vi "ACT_Loop.vi"() -> ()   [LabVIEW 2023, in "Swerve-SteerSRX-DriveSpark-AbsAnalog_ACT.lvlib"]
uses:
  Swerve-SteerSRX-DriveSpark-AbsAnalog_ACT.lvlib
  Cluster_CMD_ACT_Data.ctl
  ENUM_CMD_Mode Select.ctl
  Shared Code/TypeDefs/Cluster_CMD_Direction Data.ctl
  Shared Code/TypeDefs/Cluster_Module Velocity-Direction-Rotations.ctl
  Shared Code/TypeDefs/Level_Velocity plus-minus 1.ctl
  Shared Code/TypeDefs/Dial_Compase heading unit circle CCW positive.ctl
  Shared Code/TypeDefs/Cluster_X-Y.ctl
  Cluster_HW Output Values.ctl
  Shared Code/TypeDefs/Cluster_Swerve 4 Steer and Velocity.ctl
  Cluster_System Output Data.ctl
  Cluster_System Config_Values.ctl
  Shared Code/TypeDefs/Cluster_SW PID Config.ctl
  Shared Code/TypeDefs/Cluster_PID Gains.ctl
  Shared Code/TypeDefs/Cluster_High-Low.ctl
  Type Defs/Cluster_Length and Width.ctl
  Shared Code/TypeDefs/Cluster_Config_Swerve_Drive Param.ctl
  Shared Code/TypeDefs/Cluster_Config_Swerve_Steer Parm.ctl
  Cluster_Config Specific HW Values.ctl
  Cluster_Config Specific Data.ctl
  Shared Code/TypeDefs/ENUM_Module Position.ctl
  Cluster_Config Steer HW Values.ctl
  Shared Code/TypeDefs/Cluster_Config SRX Motor Output.ctl
  <vilib>/Rock Robotics/WPI/ThirdParty/Phoenix-LabVIEW/Motor Controller/Controls/CTRE_Phoenix_MotorControl_NeutralMode.ctl
  Shared Code/TypeDefs/Cluster_FWD  REV Values.ctl
  Shared Code/TypeDefs/Cluster_SRX SLOT PID Config.ctl
  Shared Code/TypeDefs/Cluster_SRX Motion Magic Parameters.ctl
  Cluster_Config Drive HW Values.ctl
  Shared Code/TypeDefs/Cluster_SparkMax Config_Motor Output.ctl
  <vilib>/Rock Robotics/WPI/ThirdParty/REV Robotics/REVLib/Typedef/Spark MAX Idle Mode.ctl
  Shared Code/TypeDefs/Cluster_Spark MAX Config_SLOT PID Config.ctl
  Shared Code/TypeDefs/Cluster_SparkMax Config_Smart Motion Parameters.ctl
  ENUM_ACT_State.ctl
  <vilib>/Rock Robotics/WPI/ThirdParty/Phoenix-LabVIEW/Motor Controller/Controls/CTRE_Phoenix_MotorControl_ControlMode.ctl
  <vilib>/Rock Robotics/WPI/MotorControl/WPI_MotorControlDeviceRef.ctl
  <vilib>/Rock Robotics/WPI/MotorControl/WPI_MotorControlType.ctl
  <vilib>/Rock Robotics/SystemInterfaces/DIO/FPGA_DIOPWMChannel.ctl
  <vilib>/Rock Robotics/WPI/PWM/WPI_PWMDeadband.ctl
  <vilib>/Rock Robotics/SystemInterfaces/DIO/FPGA_DIOChannel.ctl
  ENUM_ACT_Action.ctl
  4f1f8321-3dc8-4b28-8619-20673fc77ec2.vi
  cbff3d61-3b62-444e-9844-795ae03579cd.vi
  089052c0-d540-4a78-a5cc-aeb70dbb496b.vi
  6201c2b1-dcd8-4430-86f1-9b4ee56c7753.vi
  b5508d6c-c1cc-4273-80c5-2077d34e1483.vi
  5f725c2a-0ce1-4524-8967-e83b15fdce90.vi
  bd5da564-2e8e-4505-86fc-30918feadaa2.vi
  8beda75f-c59a-4462-acc7-7c37ceab3777.vi
  47a9b741-f4a3-48b6-ae85-4ba2e502368e.vi
  e2e8a241-7810-4d95-85fd-17f3a55957a8.vi
  80d407e5-f582-430c-986f-ecd413765478.vi
  573e44c0-11f4-4bd9-ad56-904ec25dba75.vi
  e7494af9-f670-4352-9dfa-ae6ce50709ea.vi
  <vilib>/Utility/error.llb/Trim Whitespace.vi
  5f725c2a-0ce1-4524-8967-e83b15fdce90.vi/958b2683-dd4b-41b7-8ed1-41c95f63cef0.vi
  5f725c2a-0ce1-4524-8967-e83b15fdce90.vi/95f5fa9b-6175-4b34-88ee-cece92c38279.vi
  bd5da564-2e8e-4505-86fc-30918feadaa2.vi/958b2683-dd4b-41b7-8ed1-41c95f63cef0.vi
  bd5da564-2e8e-4505-86fc-30918feadaa2.vi/95f5fa9b-6175-4b34-88ee-cece92c38279.vi
  8beda75f-c59a-4462-acc7-7c37ceab3777.vi/958b2683-dd4b-41b7-8ed1-41c95f63cef0.vi
  8beda75f-c59a-4462-acc7-7c37ceab3777.vi/95f5fa9b-6175-4b34-88ee-cece92c38279.vi
  47a9b741-f4a3-48b6-ae85-4ba2e502368e.vi/958b2683-dd4b-41b7-8ed1-41c95f63cef0.vi
  47a9b741-f4a3-48b6-ae85-4ba2e502368e.vi/95f5fa9b-6175-4b34-88ee-cece92c38279.vi
  e2e8a241-7810-4d95-85fd-17f3a55957a8.vi/958b2683-dd4b-41b7-8ed1-41c95f63cef0.vi
  e2e8a241-7810-4d95-85fd-17f3a55957a8.vi/95f5fa9b-6175-4b34-88ee-cece92c38279.vi
  80d407e5-f582-430c-986f-ecd413765478.vi/958b2683-dd4b-41b7-8ed1-41c95f63cef0.vi
  80d407e5-f582-430c-986f-ecd413765478.vi/95f5fa9b-6175-4b34-88ee-cece92c38279.vi
  573e44c0-11f4-4bd9-ad56-904ec25dba75.vi/958b2683-dd4b-41b7-8ed1-41c95f63cef0.vi
  573e44c0-11f4-4bd9-ad56-904ec25dba75.vi/95f5fa9b-6175-4b34-88ee-cece92c38279.vi
  e7494af9-f670-4352-9dfa-ae6ce50709ea.vi/958b2683-dd4b-41b7-8ed1-41c95f63cef0.vi
  e7494af9-f670-4352-9dfa-ae6ce50709ea.vi/95f5fa9b-6175-4b34-88ee-cece92c38279.vi
  <vilib>/Utility/error.llb/Trim Whitespace One-Sided.vi
  5f725c2a-0ce1-4524-8967-e83b15fdce90.vi/95f5fa9b-6175-4b34-88ee-cece92c38279.vi/1c6bd52c-bbca-4d4a-a290-93ea2703fded.vi
  5f725c2a-0ce1-4524-8967-e83b15fdce90.vi/95f5fa9b-6175-4b34-88ee-cece92c38279.vi/47c2b0d5-b5fa-444e-9535-611565d375db.vi
  bd5da564-2e8e-4505-86fc-30918feadaa2.vi/95f5fa9b-6175-4b34-88ee-cece92c38279.vi/1c6bd52c-bbca-4d4a-a290-93ea2703fded.vi
  bd5da564-2e8e-4505-86fc-30918feadaa2.vi/95f5fa9b-6175-4b34-88ee-cece92c38279.vi/47c2b0d5-b5fa-444e-9535-611565d375db.vi
  8beda75f-c59a-4462-acc7-7c37ceab3777.vi/95f5fa9b-6175-4b34-88ee-cece92c38279.vi/1c6bd52c-bbca-4d4a-a290-93ea2703fded.vi
  8beda75f-c59a-4462-acc7-7c37ceab3777.vi/95f5fa9b-6175-4b34-88ee-cece92c38279.vi/47c2b0d5-b5fa-444e-9535-611565d375db.vi
  47a9b741-f4a3-48b6-ae85-4ba2e502368e.vi/95f5fa9b-6175-4b34-88ee-cece92c38279.vi/1c6bd52c-bbca-4d4a-a290-93ea2703fded.vi
  47a9b741-f4a3-48b6-ae85-4ba2e502368e.vi/95f5fa9b-6175-4b34-88ee-cece92c38279.vi/47c2b0d5-b5fa-444e-9535-611565d375db.vi
  e2e8a241-7810-4d95-85fd-17f3a55957a8.vi/95f5fa9b-6175-4b34-88ee-cece92c38279.vi/1c6bd52c-bbca-4d4a-a290-93ea2703fded.vi
  e2e8a241-7810-4d95-85fd-17f3a55957a8.vi/95f5fa9b-6175-4b34-88ee-cece92c38279.vi/47c2b0d5-b5fa-444e-9535-611565d375db.vi
  80d407e5-f582-430c-986f-ecd413765478.vi/95f5fa9b-6175-4b34-88ee-cece92c38279.vi/1c6bd52c-bbca-4d4a-a290-93ea2703fded.vi
  80d407e5-f582-430c-986f-ecd413765478.vi/95f5fa9b-6175-4b34-88ee-cece92c38279.vi/47c2b0d5-b5fa-444e-9535-611565d375db.vi
  573e44c0-11f4-4bd9-ad56-904ec25dba75.vi/95f5fa9b-6175-4b34-88ee-cece92c38279.vi/1c6bd52c-bbca-4d4a-a290-93ea2703fded.vi
  573e44c0-11f4-4bd9-ad56-904ec25dba75.vi/95f5fa9b-6175-4b34-88ee-cece92c38279.vi/47c2b0d5-b5fa-444e-9535-611565d375db.vi
  e7494af9-f670-4352-9dfa-ae6ce50709ea.vi/95f5fa9b-6175-4b34-88ee-cece92c38279.vi/1c6bd52c-bbca-4d4a-a290-93ea2703fded.vi
  e7494af9-f670-4352-9dfa-ae6ce50709ea.vi/95f5fa9b-6175-4b34-88ee-cece92c38279.vi/47c2b0d5-b5fa-444e-9535-611565d375db.vi
  RoboRIO Utilities/Global_STOP.vi
  Global_CMD_ACT_Data In.vi
  PigeonIMU/Global_SEN_Data Out.vi
  Global_ACT_Data Out.vi
  <vilib>/Utility/Data Type/Get Type Information.vi
  Shared Code/Utility/RWA/RWA/File/RWA_PC FIle Read String.vi
  Shared Code/Utility/RWA/RWA/Read Write Anything/RWA_File String.vi
  Shared Code/Utility/RWA/RWA/File/RWA_PC File Write String.vi
  <vilib>/Comparison/Equal/Equal Functor/Equal Functor.lvclass
  PigeonIMU/PigeonIMU_SEN_ts.lvlib
panel:
  in  "Set Steer Start Values":bool
  in  "Config Drive":T1={"Drive HW Ver"=0, "SparkMax Output"={"Motor Invert"=FALSE, "Ramp Rate OL (S)"=1.0, "Dead Band"=0.0, "Idle Mode"=enum."Coast"}, "Slot 0 CL"={"Gains"={"P"=0.1, "I"=0.0, "D"=0.0, "F"=0.0}, "I Zone"=0.0, "Peak Out -1 0 1"={"High"=0.0, "Low"=0.0}, "Max I Accu"=0.0}, "Slot 0 SM"={"Max Velocity"=0.0, "Max Acceleration"=0.0, "Allowed CL Error"=0.0, "Min Velocity Output"=0.0}} {"Slot 0 CL"."Gains"."F" format="%#.8f"; "Slot 0 CL"."Gains"."D" format="%#.8f"; "Slot 0 CL"."Gains"."I" format="%#.8f"; "Slot 0 CL"."Gains"."P" format="%#.8f"; "Slot 0 CL"."Peak Out -1 0 1"."Low" format="%#.8f"; "Slot 0 CL"."Peak Out -1 0 1"."High" format="%#.8f"}
  in  "Config Steer":T8={"Steer HW Ver"=0, "SRX Output"={"Neutral"=enum."Override to Coast", "Max"={"FWD"=1.0, "REV"=-1.0}, "Min"={"FWD"=0.0, "REV"=0.0}, "OL Ramp Rate (S)"=0.0, "Dead Band"=0.0, "CL Ramp Rate (S)"=0.0}, "Slot 0 CL"={"Gains"={"P"=1.0, "I"=0.01, "D"=0.0, "F"=0.0}, "Error Allowed"=0.0, "I Zone"=10000.0, "Peak Out 0-1"=1.0, "Max I Accu"=-1000.0}, "Slot 0 MM"={"Cruise Velocity"=5000, "Acceleration"=5000}} {"Slot 0 CL"."Gains"."F" format="%#.8f"; "Slot 0 CL"."Gains"."D" format="%#.8f"; "Slot 0 CL"."Gains"."I" format="%#.8f"; "Slot 0 CL"."Gains"."P" format="%#.8f"; "SRX Output"."Min"."REV" format="%.2f"; "SRX Output"."Min"."FWD" format="%.2f"; "SRX Output"."Max"."REV" format="%.2f"; "SRX Output"."Max"."FWD" format="%.2f"}
  in  "Config Specific":T14={"Specific HW Ver"=0, "Specific Data"=[{"Motor Pos"=enum."Left-Front", "CAN Bus"="", "Drive ID"=0, "Steer ID"=0, "Encoder Start Value"=0.0}, {"Motor Pos"=enum."Right-Front", "CAN Bus"="", "Drive ID"=0, "Steer ID"=0, "Encoder Start Value"=0.0}, {"Motor Pos"=enum."Right-Back", "CAN Bus"="", "Drive ID"=0, "Steer ID"=0, "Encoder Start Value"=0.0}, {"Motor Pos"=enum."Left-Back", "CAN Bus"="", "Drive ID"=0, "Steer ID"=0, "Encoder Start Value"=0.0}]}
  in  "CMD Override":enum32{"None", "Mode 2", "Mode 1", "STOP"}(tab)
  in  "Mode 2 Data":dbl(slide) scale=-0.2..0.2
  in  "Mode 1 Data":i32
  in  "GO":bool
  out "Current Time":timestamp
  in  "Config System":T17={"System Ver"=0, "Auto Angle PID"={"Gains"={"P"=0.1, "I"=0.0, "D"=0.0, "F"=0.0}, "Error Allowed"={"High"=0.0, "Low"=0.0}, "I Zone"={"High"=0.0, "Low"=0.0}, "Peak Out 0-1"={"High"=0.0, "Low"=0.0}, "Max I Accu"={"High"=0.0, "Low"=0.0}}, "Frame"={"Length"=33.0, "Width"=18.0}, "Drive Data"={"CPR"=14.0, "RevMotor/Wheel"=6.67, "Wheel Diameter (in)"=4.0}, "Speed Full Scale"=5000.0, "Steer Data"={"CPR"=1024.0}} {"Auto Angle PID"."Max I Accu"."Low" format="%#.8f"; "Auto Angle PID"."Max I Accu"."High" format="%#.8f"; "Auto Angle PID"."Gains"."F" format="%#.8f"; "Auto Angle PID"."Gains"."D" format="%#.8f"; "Auto Angle PID"."Gains"."I" format="%#.8f"; "Auto Angle PID"."Gains"."P" format="%#.8f"; "Auto Angle PID"."Error Allowed"."Low" format="%#.8f"; "Auto Angle PID"."Error Allowed"."High" format="%#.8f"; "Auto Angle PID"."I Zone"."Low" format="%#.8f"; "Auto Angle PID"."I Zone"."High" format="%#.8f"; "Auto Angle PID"."Peak Out 0-1"."Low" format="%#.8f"; "Auto Angle PID"."Peak Out 0-1"."High" format="%#.8f"}
  out "System Config":T22
  out "Sensor Read time":dbl format="%.3g"
  out "HW Output":T23 {"Swerve Read"."Back Right"."Angle" scale format="%.3f"; "Swerve Read"."Back Right"."Velocity" scale=-1.0..1.0 scale format="%.1f"; "Swerve Read"."Back Left"."Angle" scale format="%.3f"; "Swerve Read"."Back Left"."Velocity" scale=-1.0..1.0 scale format="%.1f"; "Swerve Read"."Front Left"."Angle" scale format="%.3f"; "Swerve Read"."Front Left"."Velocity" scale=-1.0..1.0 scale format="%.1f"; "Swerve Read"."Front Right"."Angle" scale format="%.3f"; "Swerve Read"."Front Right"."Velocity" scale=-1.0..1.0 scale format="%.1f"; "Pigeon Heading" scale format="%.3f"}
  in  "Read Saved Config":bool
  in  "Update Config":bool
  out "CMD":T28 {"Target Auto Angle" scale format="%.3f"; "Direction"."Rotate(Yaw) CCW 1 CW -1" scale=1.0..-1.0; "Direction"."Traverse"."Angle" scale format="%.3f"; "Direction"."Traverse"."Velocity" scale=-1.0..1.0 scale format="%.1f"}
  out "Cycle Time (S)":dbl format="%.3g"
  # "STOP"
  # "\"Front\" of Robot"
  # "Index 1"
  # "Index 0"
  # "Index 3"
  # "Index 2"
  # "Right Hand Rule"
  # "X"
  # "+CCW"
  # "Y"
  # "(0,0)"
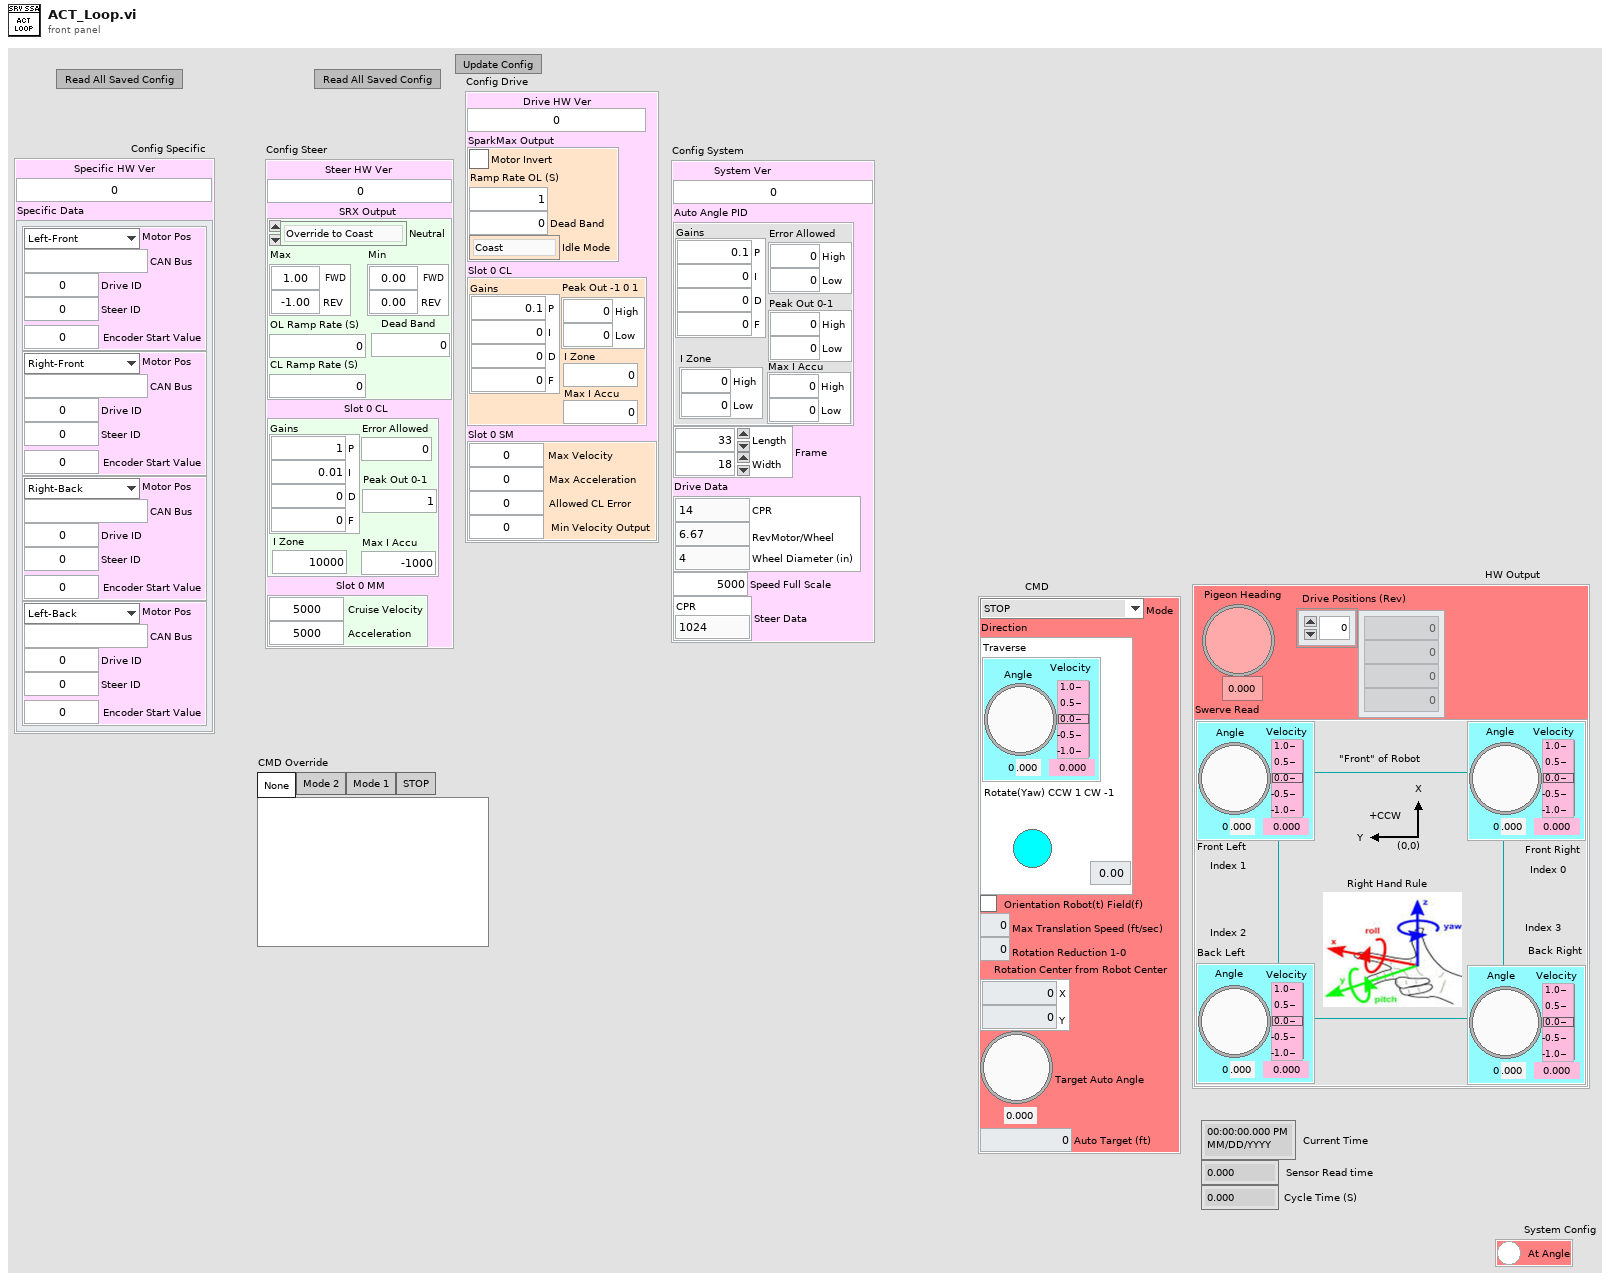
[diagram p1: front panel]
types:
  T1 = typedef "Swerve-SteerSRX-DriveSpark-AbsAnalog_ACT.lvlib/Cluster_Config Drive HW Values.ctl" = cluster{"Drive HW Ver":u64, "SparkMax Output":T2, "Slot 0 CL":T4, "Slot 0 SM":T7}
  T2 = typedef "Cluster_SparkMax Config_Motor Output.ctl" = cluster{"Motor Invert":bool, "Ramp Rate OL (S)":dbl, "Dead Band":dbl, "Idle Mode":T3}
  T3 = typedef "Spark MAX Idle Mode.ctl" = enum16{"Coast", "Brake"}
  T4 = typedef "Cluster_Spark MAX Config_SLOT PID Config.ctl" = cluster{"Gains":T5, "I Zone":dbl, "Peak Out -1 0 1":T6, "Max I Accu":dbl}
  T5 = typedef "Cluster_PID Gains.ctl" = cluster{"P":dbl, "I":dbl, "D":dbl, "F":dbl}
  T6 = typedef "Cluster_High-Low.ctl" = cluster{"High":dbl, "Low":dbl}
  T7 = typedef "Cluster_SparkMax Config_Smart Motion Parameters.ctl" = cluster{"Max Velocity":dbl, "Max Acceleration":dbl, "Allowed CL Error":dbl, "Min Velocity Output":dbl}
  T8 = typedef "Swerve-SteerSRX-DriveSpark-AbsAnalog_ACT.lvlib/Cluster_Config Steer HW Values.ctl" = cluster{"Steer HW Ver":u64, "SRX Output":T9, "Slot 0 CL":T12, "Slot 0 MM":T13}
  T9 = typedef "Cluster_Config SRX Motor Output.ctl" = cluster{"Neutral":T10, "Max":T11, "Min":T11, "OL Ramp Rate (S)":dbl, "Dead Band":dbl, "CL Ramp Rate (S)":dbl}
  T10 = typedef "CTRE_Phoenix_MotorControl_NeutralMode.ctl" = enum8{"EEPROMSetting", "Override to Coast", "Override to Brake"}
  T11 = typedef "Cluster_FWD  REV Values.ctl" = cluster{"FWD":dbl, "REV":dbl}
  T12 = typedef "Cluster_SRX SLOT PID Config.ctl" = cluster{"Gains":T5, "Error Allowed":dbl, "I Zone":dbl, "Peak Out 0-1":dbl, "Max I Accu":dbl}
  T13 = typedef "Cluster_SRX Motion Magic Parameters.ctl" = cluster{"Cruise Velocity":i32, "Acceleration":i32}
  T14 = typedef "Swerve-SteerSRX-DriveSpark-AbsAnalog_ACT.lvlib/Cluster_Config Specific HW Values.ctl" = cluster{"Specific HW Ver":u64, "Specific Data":T15[]}
  T15 = typedef "Swerve-SteerSRX-DriveSpark-AbsAnalog_ACT.lvlib/Cluster_Config Specific Data.ctl" = cluster{"Motor Pos":T16, "CAN Bus":string, "Drive ID":u8, "Steer ID":u8, "Encoder Start Value":dbl}
  T16 = typedef "ENUM_Module Position.ctl" = enum16{"Left-Front", "Right-Front", "Left-Back", "Right-Back"}
  T17 = typedef "Swerve-SteerSRX-DriveSpark-AbsAnalog_ACT.lvlib/Cluster_System Config_Values.ctl" = cluster{"System Ver":u64, "Auto Angle PID":T18, "Frame":T19, "Drive Data":T20, "Speed Full Scale":dbl, "Steer Data":T21}
  T18 = typedef "Cluster_SW PID Config.ctl" = cluster{"Gains":T5, "Error Allowed":T6, "I Zone":T6, "Peak Out 0-1":T6, "Max I Accu":T6}
  T19 = typedef "Cluster_Length and Width.ctl" = cluster{"Length":dbl, "Width":dbl}
  T20 = typedef "Cluster_Config_Swerve_Drive Param.ctl" = cluster{"CPR":dbl, "RevMotor/Wheel":dbl, "Wheel Diameter (in)":dbl}
  T21 = typedef "Cluster_Config_Swerve_Steer Parm.ctl" = cluster{"CPR":dbl}
  T22 = typedef "Swerve-SteerSRX-DriveSpark-AbsAnalog_ACT.lvlib/Cluster_System Output Data.ctl" = cluster{"At Angle":bool}
  T23 = typedef "Swerve-SteerSRX-DriveSpark-AbsAnalog_ACT.lvlib/Cluster_HW Output Values.ctl" = cluster{"Pigeon Heading":T24, "Swerve Read":T25, "Drive Positions (Rev)":dbl[]}
  T24 = typedef "Dial_Compase heading unit circle CCW positive.ctl" = dbl
  T25 = typedef "Cluster_Swerve 4 Steer and Velocity.ctl" = cluster{"Front Right":T26, "Front Left":T26, "Back Left":T26, "Back Right":T26}
  T26 = typedef "Cluster_Module Velocity-Direction-Rotations.ctl" = cluster{"Velocity":T27, "Angle":T24, "Rotations Count":dbl}
  T27 = typedef "Level_Velocity plus-minus 1.ctl" = dbl
  T28 = typedef "Swerve-SteerSRX-DriveSpark-AbsAnalog_ACT.lvlib/Cluster_CMD_ACT_Data.ctl" = cluster{"Mode":T29, "Direction":T30, "Orientation Robot(t) Field(f)":bool, "Max Translation Speed (ft/sec)":dbl, "Rotation Reduction 1-0":dbl, "Rotation Center from Robot Center":T31, "Target Auto Angle":T24, "Auto Target (ft)":dbl}
  T29 = typedef "Swerve-SteerSRX-DriveSpark-AbsAnalog_ACT.lvlib/ENUM_CMD_Mode Select.ctl" = enum16{"STOP", "Move", "Turret Manual", "Trans Manual Angle Auto", "Turret Auto Angle"}
  T30 = typedef "Cluster_CMD_Direction Data.ctl" = cluster{"Traverse":T26, "Rotate(Yaw) CCW 1 CW -1":dbl}
  T31 = typedef "Cluster_X-Y.ctl" = cluster{"X":dbl, "Y":dbl}
  T32 = typedef "WPI_MotorControlDeviceRef.ctl" = cluster{"DeviceStatus":errorcluster, "Type":T33, "PWM":cluster{"PWM Channel":T34, "DeadBand":T35}, "CAN":cluster{"Device Number":u8, "SetOutput VI Ref":variant, "GetOutput VI Ref":variant, "Enable VI Ref":variant, "Disable VI Ref":variant, "Data":variant}, "Invert":bool, "DIO PWM":cluster{"PWM \"Enable\" Channel":T34, "DIOChannel":T36, "PWM Rate":dbl}}
  T33 = typedef "WPI_MotorControlType.ctl" = enum16{"PWM", "CAN", "DIO PWM"}
  T34 = typedef "FPGA_DIOPWMChannel.ctl" = enum8{"PWM 0", "PWM 1", "PWM 2", "PWM 3", "PWM 4", "PWM 5", "PWM 6", "PWM 7", "PWM 8", "PWM 9", "PWM MXP 0", "PWM MXP 1", "PWM MXP 2", "PWM MXP 3", "PWM MXP 4", "PWM MXP 5", "PWM MXP 6", "PWM MXP 7", "PWM MXP 8", "PWM MXP 9", "Invalid"}
  T35 = typedef "WPI_PWMDeadband.ctl" = cluster{"Name":string, "maxPositivePwm":i32, "minPositivePwm":i32, "centerPwm":i32, "maxNegativePwm":i32, "minNegativePwm":i32, "angularRange":u16}
  T36 = typedef "FPGA_DIOChannel.ctl" = enum8{"DIO 0", "DIO 1", "DIO 2", "DIO 3", "DIO 4", "DIO 5", "DIO 6", "DIO 7", "DIO 8", "DIO 9", "DIO MXP 0", "DIO MXP 1", "DIO MXP 2", "DIO MXP 3", "DIO MXP 4", "DIO MXP 5", "DIO MXP 6", "DIO MXP 7", "DIO MXP 8", "DIO MXP 9", "DIO MXP 10", "DIO MXP 11", "DIO MXP 12", "DIO MXP 13", "DIO MXP 14", "DIO MXP 15", "SPI Port CS1", "SPI Port CS2", "SPI Port CS3", "SPI Port MISO", "SPI Port MOSI", "Invalid"}
  T37 = typedef "CTRE_Phoenix_MotorControl_ControlMode.ctl" = u16
  T38 = typedef "Swerve-SteerSRX-DriveSpark-AbsAnalog_ACT.lvlib/ENUM_ACT_State.ctl" = enum16{"Startup", "Configuring", "Stopping", "Moving Mode 1", "Moving Mode 2", "Shutdown", "Initializing HW"}
  T39 = cluster{"Motor List":T16[], "Team Folder":path, "FX Ref":T32, "Steer Refs":T32[], "Drive Refs":T32[], "State":T38, "Previous State":T38, "Current Time":timestamp, "Previous Time":timestamp, "Start Time":timestamp, "Target Time (ms)":u32, "Cycle Time(S)":dbl, "Update Display":bool, "ACT Input":T28, "Config System":T17, "Max # Of Config Tries":i32, "HW Out":T23, "System Output":T22, "CAN Timeout":u32, "FX Mode":T37, "FX Set Value":dbl, "Config Specific":T14, "Swerve Set":T25, "New Cmd":bool, "Config Steer":T8, "Config Drive":T1, "HW OPEN":bool, "Steer Change":bool, "Drive Change":bool, "Specific Change":bool, "System Change":bool}
  T40 = typedef "Swerve-SteerSRX-DriveSpark-AbsAnalog_ACT.lvlib/ENUM_ACT_Action.ctl" = enum16{"No Action", "Reset Time", "Reset All", "Open HW References", "Control FX Stop", "Control FX Mode 1", "Control FX Mode 2", "Set Robot Start Position", "Config HW Steer Set", "Config HW Steer Get", "Config HW Steer Save", "Config HW Steer Read", "Config HW Drive Set", "Config HW Drive Get", "Config HW Drive Save", "Config HW Drive Read", "Config HW Specific Set", "Config HW Specific Get", "Config HW Specific Save", "Config HW Specific Read", "Config System Save", "Config System Read", "Config From FP", "Start HW Steer Set", "Default HW Steer Set", "Defalut HW Drive Set"}
  T41 = cluster{"[0]":T26, "[1]":T26, "[2]":T26, "[3]":T26}
  T42 = typedef "Cluster_Unity Yaw-Pitch-Roll.ctl" = cluster{"Yaw":T24, "Pitch":T24, "Roll":T24}
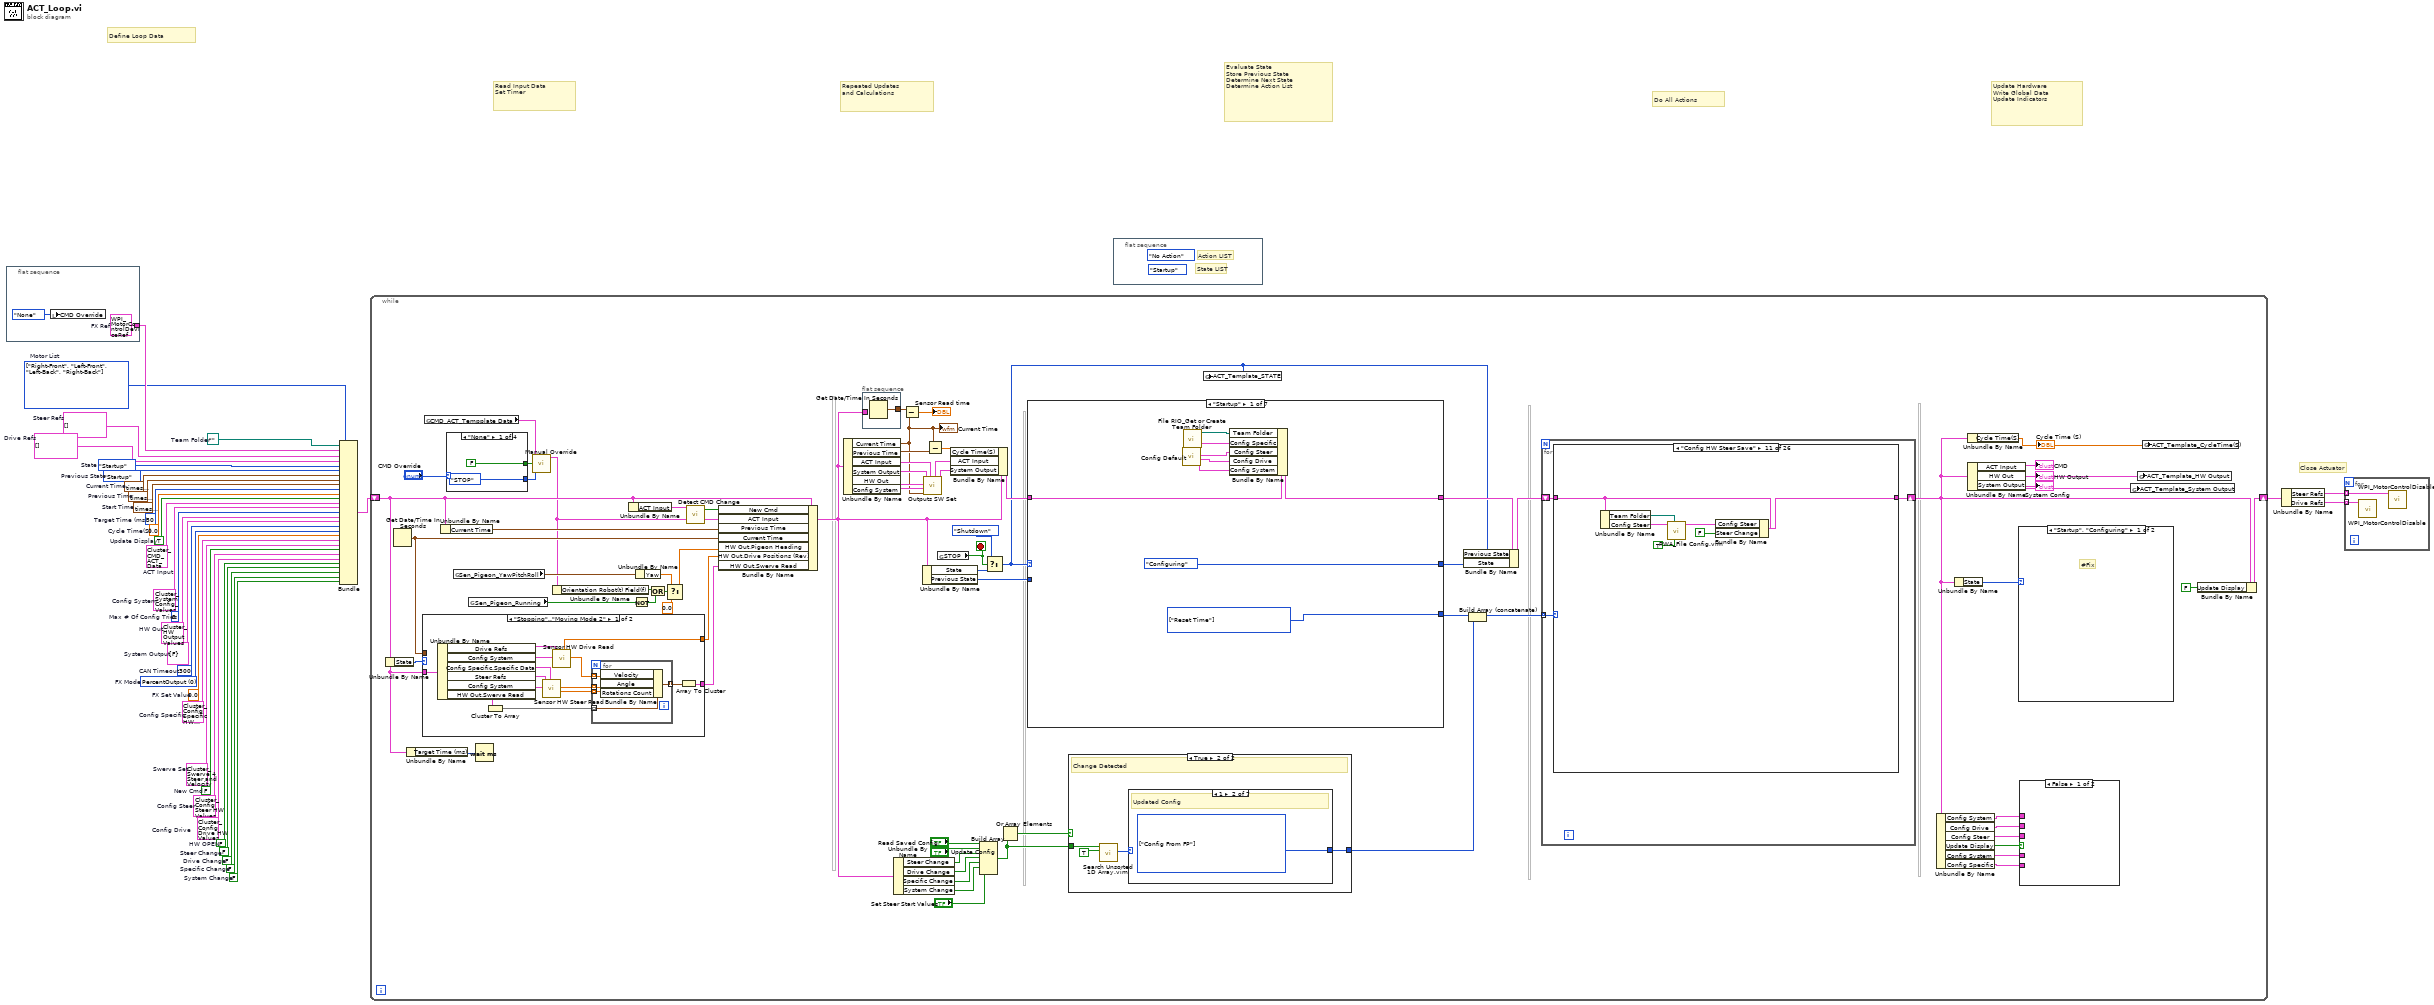
[diagram p0: block diagram]
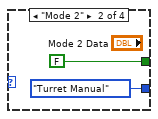
[diagram p2: hidden frame]
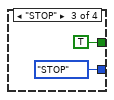
[diagram p3: hidden frame]
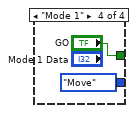
[diagram p4: hidden frame]
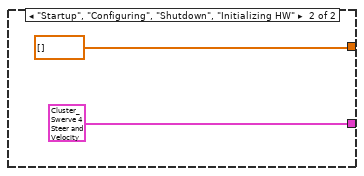
[diagram p5: hidden frame]
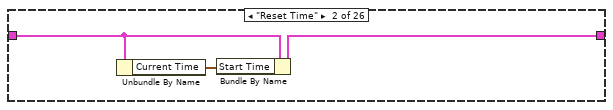
[diagram p7: hidden frame]
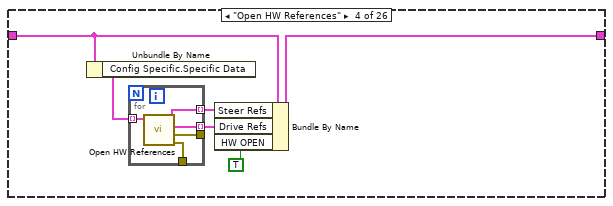
[diagram p9: hidden frame]
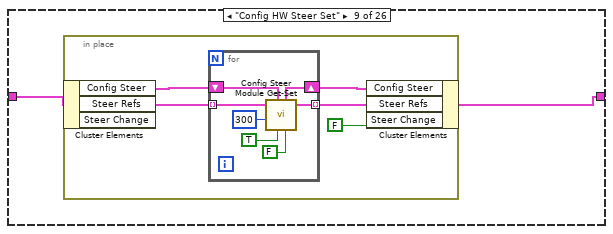
[diagram p14: hidden frame]
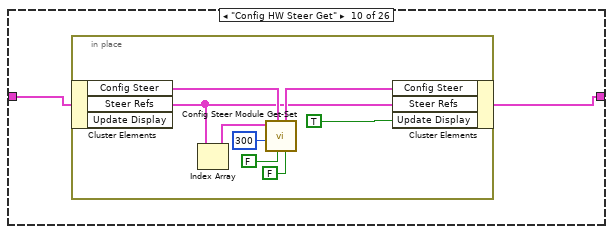
[diagram p15: hidden frame]
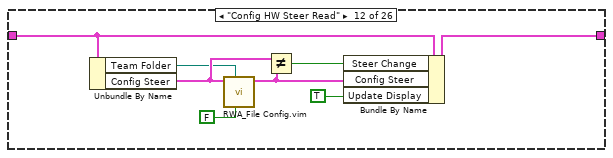
[diagram p16: hidden frame]
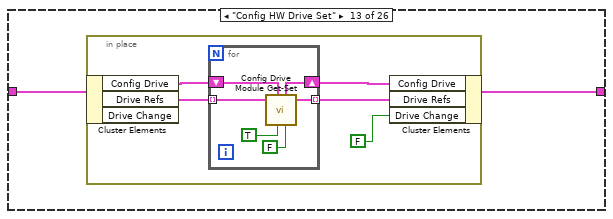
[diagram p17: hidden frame]
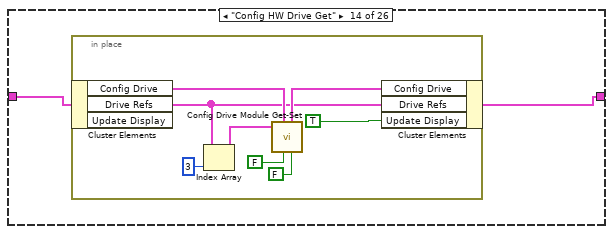
[diagram p18: hidden frame]
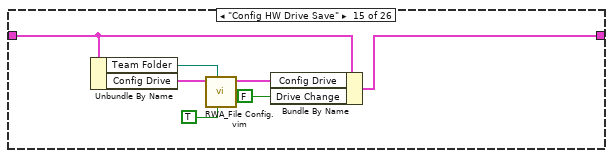
[diagram p19: hidden frame]
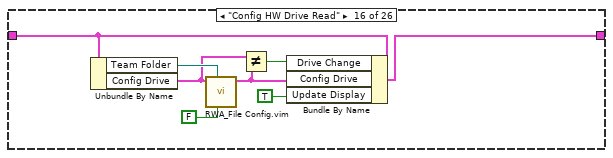
[diagram p20: hidden frame]
diagram:
  w1 = FALSE  # System Change
  w2 = FALSE  # Specific Change
  w3 = FALSE  # Drive Change
  w4 = FALSE  # Steer Change
  w5 = FALSE  # HW OPEN
  w7 = T8 {"Steer HW Ver"=0, "SRX Output"={"Neutral"=enum."Override to Coast", "Max"={"FWD"=1.0, "REV"=-1.0}, "Min"={"FWD"=0.0, "REV"=0.0}, "OL Ramp Rate (S)"=0.0, "Dead Band"=0.0, "CL Ramp Rate (S)"=0.0}, "Slot 0 CL"={"Gains"={"P"=1.0, "I"=0.01, "D"=0.0, "F"=0.0}, "Error Allowed"=0.0, "I Zone"=10000.0, "Peak Out 0-1"=1.0, "Max I Accu"=-1000.0}, "Slot 0 MM"={"Cruise Velocity"=5000, "Acceleration"=5000}}  # Config Steer
  w6 = T1 {"Drive HW Ver"=0, "SparkMax Output"={"Motor Invert"=FALSE, "Ramp Rate OL (S)"=1.0, "Dead Band"=0.0, "Idle Mode"=enum."Coast"}, "Slot 0 CL"={"Gains"={"P"=0.1, "I"=0.0, "D"=0.0, "F"=0.0}, "I Zone"=0.0, "Peak Out -1 0 1"={"High"=0.0, "Low"=0.0}, "Max I Accu"=0.0}, "Slot 0 SM"={"Max Velocity"=0.0, "Max Acceleration"=0.0, "Allowed CL Error"=0.0, "Min Velocity Output"=0.0}}  # Config Drive
  w8 = FALSE  # New Cmd
  w9 = path ""  # Team Folder
  w11 = T25 {"Front Right"={"Velocity"=0.0, "Angle"=0.0, "Rotations Count"=0.0}, "Front Left"={"Velocity"=0.0, "Angle"=0.0, "Rotations Count"=0.0}, "Back Left"={"Velocity"=0.0, "Angle"=0.0, "Rotations Count"=0.0}, "Back Right"={"Velocity"=0.0, "Angle"=0.0, "Rotations Count"=0.0}}  # Swerve Set
  w12 = T16[] [enum."Right-Front", enum."Left-Front", enum."Left-Back", enum."Right-Back"] items=["Left-Front", "Right-Front", "Left-Back", "Right-Back"]  # Motor List
  w15 = T32[] []  # Steer Refs
  w14 = T32[] []  # Drive Refs
  w16 = T14 {"Specific HW Ver"=0, "Specific Data"=[{"Motor Pos"=enum."Left-Front", "CAN Bus"="", "Drive ID"=0, "Steer ID"=0, "Encoder Start Value"=0.0}, {"Motor Pos"=enum."Right-Front", "CAN Bus"="", "Drive ID"=0, "Steer ID"=0, "Encoder Start Value"=0.0}, {"Motor Pos"=enum."Right-Back", "CAN Bus"="", "Drive ID"=0, "Steer ID"=0, "Encoder Start Value"=0.0}, {"Motor Pos"=enum."Left-Back", "CAN Bus"="", "Drive ID"=0, "Steer ID"=0, "Encoder Start Value"=0.0}]}  # Config Specific
  w22 = T22 {"At Angle"=FALSE}  # System Output
  w24 = T17 {"System Ver"=0, "Auto Angle PID"={"Gains"={"P"=0.2, "I"=0.0, "D"=0.0, "F"=0.0}, "Error Allowed"={"High"=0.0, "Low"=0.0}, "I Zone"={"High"=0.0, "Low"=0.0}, "Peak Out 0-1"={"High"=0.0, "Low"=0.0}, "Max I Accu"={"High"=0.0, "Low"=0.0}}, "Frame"={"Length"=33.0, "Width"=18.0}, "Drive Data"={"CPR"=14.0, "RevMotor/Wheel"=6.67, "Wheel Diameter (in)"=4.0}, "Speed Full Scale"=5000.0, "Steer Data"={"CPR"=1024.0}}  # Config System
  w23 = T23 {"Pigeon Heading"=0.0, "Swerve Read"={"Front Right"={"Velocity"=0.0, "Angle"=0.0, "Rotations Count"=0.0}, "Front Left"={"Velocity"=0.0, "Angle"=0.0, "Rotations Count"=0.0}, "Back Left"={"Velocity"=0.0, "Angle"=0.0, "Rotations Count"=0.0}, "Back Right"={"Velocity"=0.0, "Angle"=0.0, "Rotations Count"=0.0}}, "Drive Positions (Rev)"=[]}  # HW Out
  w19 = 0.0  # FX Set Value
  w20 = T37 0 items=["PercentOutput"=0, "Position"=1, "Velocity"=2, "Current"=3, "Follower"=5, "MotionProfile"=6, "MotionMagic"=7, "MotionProfileArc"=10, "Disabled"=15]  # FX Mode
  w18 = u32 300  # CAN Timeout
  w17 = 3  # Max # Of Config Tries
  w26 = TRUE  # Update Display
  w29 = 0.0  # Cycle Time(S)
  w30 = ENUM_ACT_State."Startup"  # Previous State
  w31 = timestamp(0 s since 1904-01-01)  # Previous Time
  w32 = u32 50  # Target Time (ms)
  w21 = T28 {"Mode"=enum."STOP", "Direction"={"Traverse"={"Velocity"=0.0, "Angle"=0.0, "Rotations Count"=0.0}, "Rotate(Yaw) CCW 1 CW -1"=0.0}, "Orientation Robot(t) Field(f)"=FALSE, "Max Translation Speed (ft/sec)"=0.0, "Rotation Reduction 1-0"=0.0, "Rotation Center from Robot Center"={"X"=0.0, "Y"=0.0}, "Target Auto Angle"=0.0, "Auto Target (ft)"=0.0}  # ACT Input
  w33 = timestamp(0 s since 1904-01-01)  # Start Time
  w34 = timestamp(0 s since 1904-01-01)  # Current Time
  w35 = ENUM_ACT_State."Startup"  # State
  # "Close Actuator"
  # "Define Loop Data"
  # "Repeated Updates\nand Calculations"
  # "Read Input Data\nSet Timer"
  # "Evaluate State\nStore Previous State\nDetermine Next State\nDetermine Action List"
  # "Do All Actions"
  # "Update Hardware\nWrite Global Data\nUpdate Indicators"
  n1 = flat-sequence {
    tunnel: [w37] -> w27
    frame #0 {
      w37 = T32 {"DeviceStatus"={"status"=FALSE, "code"=0, "source"=""}, "Type"=enum."PWM", "PWM"={"PWM Channel"=enum."PWM 1", "DeadBand"={"Name"="", "maxPositivePwm"=0, "minPositivePwm"=0, "centerPwm"=0, "maxNegativePwm"=0, "minNegativePwm"=0, "angularRange"=0}}, "CAN"={"Device Number"=0, "SetOutput VI Ref"=variant(enum8{"Percent VBus", "Current", "Speed", "Position", "Voltage"} enum."Percent VBus"), "GetOutput VI Ref"=variant(refnum<k1> refnum), "Enable VI Ref"=variant(dbl 12.0), "Disable VI Ref"=variant(enum8{"Percent VBus", "Speed", "Position", "Slave", "Unchanged / Invalid", "Voltage Compensation", "Current", "Motion Profile"} enum."Percent VBus"), "Data"=variant}, "Invert"=FALSE, "DIO PWM"={"PWM \"Enable\" Channel"=enum."Invalid", "DIOChannel"=enum."Invalid", "PWM Rate"=0.0}}  # FX Ref
      n2 = local write "CMD Override"(enum32{"None", "Mode 2", "Mode 1", "STOP"}."None" ("CMD Override")) -> ()
    }
  }
  n3 = Bundle("Motor List"=w12, "Team Folder"=w9, "FX Ref"=w27, "Steer Refs"=w15, "Drive Refs"=w14, "State"=w35, "Previous State"=w30, "Current Time"=w34, "Previous Time"=w31, "Start Time"=w33, "Target Time (ms)"=w32, "Cycle Time(S)"=w29, "Update Display"=w26, "ACT Input"=w21, "Config System"=w24, "Max # Of Config Tries"=w17, "HW Out"=w23, "System Output"=w22, "CAN Timeout"=w18, "FX Mode"=w20, "FX Set Value"=w19, "Config Specific"=w16, "Swerve Set"=w11, "New Cmd"=w8, "Config Steer"=w7, "Config Drive"=w6, "HW OPEN"=w5, "Steer Change"=w4, "Drive Change"=w3, "Specific Change"=w2, "System Change"=w1) -> (w10:T39)  [unwired: 1 in]
  n4 = while {
    shift-right: [w92] -> w28
    shift-left: w10 -> [w50]
    stop <- w103 stop-if-true
    n5 = Unbundle By Name(w50) -> ("State"=w84:T38)
    n6 = Get Date/Time In Seconds() -> (seconds since 1Jan1904=w80:timestamp)
    n7 = Unbundle By Name(w50) -> ("Target Time (ms)"=w100:u32)
    n8 = case shown="\"Stopping\"..\"Moving Mode 2\"" w84 {
      tunnel: w50 -> [w127 _]
      tunnel: w80 -> [_ _]
      tunnel: [w122 T25 {"Front Right"={"Velocity"=0.0, "Angle"=0.0, "Rotations Count"=0.0}, "Front Left"={"Velocity"=0.0, "Angle"=0.0, "Rotations Count"=0.0}, "Back Left"={"Velocity"=0.0, "Angle"=0.0, "Rotations Count"=0.0}, "Back Right"={"Velocity"=0.0, "Angle"=0.0, "Rotations Count"=0.0}} ("HW Out.Swerve Read")] -> w51
      tunnel: [w117 dbl[] [] ("Drive Positions (Rev) Out")] -> w52
      frame "Stopping".."Moving Mode 2" {
        n9 = Unbundle By Name(w127) -> ("Drive Refs"=w128:T32[], "Config System"=w125:T17, "Config Specific.Specific Data"=w126:T15[], "Steer Refs"=w129:T32[], "Config System"=w116:T17, "HW Out.Swerve Read"=w124:T25)
        n10 = Cluster To Array(cluster=w124) -> (array=w123:T26[])
        n11 = call "Sensor HW Steer Read.vi"("HW Specific Config.Specific Data"=w126, "Steer"=w116, "Steer Ref"=w129) -> ("Offsets Out"=w118:dbl[], "Angles Out"=w119:dbl[])  [unwired: 5 in, 2 out]
        n12 = call "Sensor HW Drive Read.vi"("Config HW Drive Values"=w125, "Drive Ref"=w128) -> ("Drive Velocities (0-1) Out"=w120:dbl[], "Drive Positions (Rev) Out"=w117:dbl[])  [unwired: 6 in, 2 out]
        n13 = for {
          tunnel: w123 -> [w134] mode=indexing
          tunnel: [w133] -> w121 mode=indexing
          tunnel: w120 -> [w132] mode=indexing
          tunnel: w119 -> [w131] mode=indexing
          tunnel: w118 -> [w130] mode=indexing
          n14 = Bundle By Name(cluster=w134, "Velocity"=w132, "Angle"=w131, "Rotations Count"=w130) -> (w133:T26)
        }
        n15 = Array To Cluster(array=w121) -> (cluster=w122:T41)
      }
      frame "Startup", "Configuring", "Shutdown", "Initializing HW" {
      }
    }
    n16 = global read "Global_CMD_ACT_Data In.vi" "CMD_ACT_Tempplate Data"() -> (w57:T28)
    n17 = Unbundle By Name(w50) -> ("Current Time"=w99:timestamp)
    n18 = case shown="\"None\"" "CMD Override" {
      tunnel: [FALSE ("Enable") FALSE ("Enable") TRUE ("Positon GO") "GO"] -> w67
      tunnel: [ENUM_CMD_Mode_Select."STOP" ("Override") ENUM_CMD_Mode_Select."Turret Manual" ("Override") ENUM_CMD_Mode_Select."STOP" ("Override") ENUM_CMD_Mode_Select."Move" ("Override")] -> w66
      frame "None" {
      }
      frame "Mode 2" {
      }
      frame "STOP" {
      }
      frame "Mode 1" {
      }
    }
    n19 = global read "Global_SEN_Data Out.vi" "Sen_Pigeon_YawPitchRoll"() -> (w63:T42)
    n20 = global read "Global_SEN_Data Out.vi" "Sen_Pigeon_Running"() -> (w60:bool)
    n21 = Wait (ms)(milliseconds to wait=w100) -> ()  [unwired: 1 out]
    n22 = call "Manual Override.vi"("Override"=w66, "Enable"=w67, "Auto CMD"=w57) -> ("OverRide Command Out"=w48:T28)  [unwired: 8 in]
    n23 = Unbundle By Name(w48) -> ("Orientation Robot(t) Field(f)"=w64:bool)
    n24 = Unbundle By Name(w50) -> ("ACT Input"=w49:T28)
    n25 = Not(x=w60) -> (.not. x?=w59:bool)
    n26 = Unbundle By Name(w63) -> ("Yaw"=w58:T24)
    n27 = Or(x=w64, y=w59) -> (x .or. y?=w61:bool)
    n28 = Select(t=T24 0.0, s=w61, f=w58) -> (s? t:f=w56:T24)
    n29 = call "Detect CMD Change.vi"("CMD_ACT_SwerveDrive_Data"=w48, "Preious ACT Input"=w49) -> ("New Command"=w47:bool)  [unwired: 9 in]
    n30 = Bundle By Name(cluster=w50, "New Cmd"=w47, "ACT Input"=w48, "Previous Time"=w99, "Current Time"=w80, "HW Out.Pigeon Heading"=w56, "HW Out.Drive Positions (Rev)"=w52, "HW Out.Swerve Read"=w51) -> (w43:T39)
    n31 = Unbundle By Name(w43) -> ("Current Time"=w44:timestamp, "Previous Time"=w97:timestamp, "ACT Input"=w55:T28, "System Output"=w73:T22, "HW Out"=w71:T23, "Config System"=w70:T17)
    "Current Time" <- w44
    n32 = flat-sequence {
      tunnel: [w115] -> w82
      tunnel: w43 -> [_]
      frame #0 {
        n33 = Get Date/Time In Seconds() -> (seconds since 1Jan1904=w115:timestamp)
      }
    }
    n34 = Unbundle By Name(w43) -> ("Steer Change"=w42:bool, "Drive Change"=w41:bool, "Specific Change"=w40:bool, "System Change"=w39:bool)
    n35 = Subtract(x=w82, y=w44) -> (x-y=→"Sensor Read time":dbl)
    n36 = Unbundle By Name(w43) -> ("State"=w101:T38, "Previous State"=w98:T38)
    n37 = call "Outputs SW Set.vi"("Auto CMD"=w55, "Current Time"=w44, "System Config"=w70, "Sensor Values"=w71, "SW Output"=w73) -> ("SW Output Out"=w72:T22, "Auto CMD Out"=w54:T28)  [unwired: 5 in]
    n38 = Subtract(x=w44, y=w97) -> (x-y=w95:dbl)
    n39 = global read "Global_STOP.vi" "STOP"() -> (w103:bool)
    n40 = Bundle By Name(cluster=w43, "Cycle Time(S)"=w95, "ACT Input"=w54, "System Output"=w72) -> (w96:T39)
    n41 = Build Array("Read Saved Config", "Update Config", w42, w41, w40, w39, "Set Steer Start Values") -> (w76:bool[])
    n42 = Select(t=ENUM_ACT_State."Shutdown" ("State"), s=w103, f=w101) -> (s? t:f=w65:T38)
    n43 = Or Array Elements(Boolean array=w76) -> (logical OR=w77:bool)
    n44 = case shown="\"Startup\"" w65 {
      selector: w65 -> [_ _ _ _ w433 w455 _]
      tunnel: w96 -> [w336 w350 w393 w414 w434 w456 w477]
      tunnel: [w337 w350 w392 w413 w435 w457 w477] -> w105
      tunnel: [ENUM_ACT_State."Configuring" ("State") w361 w391 w412 w437 w459 ENUM_ACT_State."Shutdown" ("State")] -> w104
      tunnel: [w339 w342 w389 w410 w432 w453 w475] -> w94
      tunnel: w98 -> [_ _ _ _ _ _ _]
      frame "Startup" {
        w339 = T40[] [enum."Reset Time"] items=["No Action", "Reset Time", "Reset All", "Open HW References", "Control FX Stop", "Control FX Mode 1", "Control FX Mode 2", "Set Robot Start Position", "Config HW Steer Set", "Config HW Steer Get", "Config HW Steer Save", "Config HW Steer Read", "Config HW Drive Set", "Config HW Drive Get", "Config HW Drive Save", "Config HW Drive Read", "Config HW Specific Set", "Config HW Specific Get", "Config HW Specific Save", "Config HW Specific Read", "Config System Save", "Config System Read", "Config From FP", "Start HW Steer Set", "Default HW Steer Set", "Defalut HW Drive Set"] ("Actions")
        n45 = call "Config Default.vi"() -> ("System Config Out"=w331:T17, "Drive Default Out"=w332:T1, "Steer Default Out"=w333:T8, "Module Specific Default Out"=w334:T14)  [unwired: 8 in]
        n46 = call "File RIO_Get or Create Team Folder.vi"() -> ("Team Files Folder"=w335:path)  [unwired: 10 in, 1 out]
        n47 = Bundle By Name(cluster=w336, "Team Folder"=w335, "Config Specific"=w334, "Config Steer"=w333, "Config Drive"=w332, "Config System"=w331) -> (w337:T39)
      }
      frame "Configuring" {
        w345 = T40[] [enum."Open HW References"] items=["No Action", "Reset Time", "Reset All", "Open HW References", "Control FX Stop", "Control FX Mode 1", "Control FX Mode 2", "Set Robot Start Position", "Config HW Steer Set", "Config HW Steer Get", "Config HW Steer Save", "Config HW Steer Read", "Config HW Drive Set", "Config HW Drive Get", "Config HW Drive Save", "Config HW Drive Read", "Config HW Specific Set", "Config HW Specific Get", "Config HW Specific Save", "Config HW Specific Read", "Config System Save", "Config System Read", "Config From FP", "Start HW Steer Set", "Default HW Steer Set", "Defalut HW Drive Set"] ("Action")
        w344 = T40[] [] items=["No Action", "Reset Time", "Reset All", "Open HW References", "Control FX Stop", "Control FX Mode 1", "Control FX Mode 2", "Set Robot Start Position", "Config HW Steer Set", "Config HW Steer Get", "Config HW Steer Save", "Config HW Steer Read", "Config HW Drive Set", "Config HW Drive Get", "Config HW Drive Save", "Config HW Drive Read", "Config HW Specific Set", "Config HW Specific Get", "Config HW Specific Save", "Config HW Specific Read", "Config System Save", "Config System Read", "Config From FP", "Start HW Steer Set", "Default HW Steer Set", "Defalut HW Drive Set"] ("Action")
        n48 = Unbundle By Name(w350) -> ("HW OPEN"=w346:bool, "Team Folder"=w341:path)
        n49 = Unbundle By Name(w350) -> ("Config Steer"=w362:T8)
        n50 = Unbundle By Name(w350) -> ("Config Specific"=w354:T14)
        n51 = Unbundle By Name(w350) -> ("Config Drive"=w357:T1)
        n52 = Unbundle By Name(w350) -> ("Config System"=w359:T17)
        n53 = call "Config_Build Name.vim"("Config First Name"=w357) -> ("Cfg file"=w356:string)  [unwired: 9 in, 1 out]
        n54 = call "Config_Build Name.vim"("Config First Name"=w362) -> ("Cfg file"=w364:string)  [unwired: 9 in, 1 out]
        n55 = call "Config_Build Name.vim"("Config First Name"=w359) -> ("Cfg file"=w360:string)  [unwired: 9 in, 1 out]
        n56 = call "Config_Build Name.vim"("Config First Name"=w354) -> ("Cfg file"=w352:string)  [unwired: 9 in, 1 out]
        n57 = Build Path(base path=w341, name or relative path=w360) -> (appended path=w358:path)
        n58 = Build Path(base path=w341, name or relative path=w356) -> (appended path=w355:path)
        n59 = Build Path(base path=w341, name or relative path=w352) -> (appended path=w353:path)
        n60 = Build Path(base path=w341, name or relative path=w364) -> (appended path=w363:path)
        n61 = call <vilib>:"Check if File or Folder Exists.vi"("path"=w358) -> ("file or folder exists?"=w349:bool)  [unwired: 8 in, 2 out]
        n62 = call <vilib>:"Check if File or Folder Exists.vi"("path"=w355) -> ("file or folder exists?"=w347:bool)  [unwired: 8 in, 2 out]
        n63 = call <vilib>:"Check if File or Folder Exists.vi"("path"=w353) -> ("file or folder exists?"=w351:bool)  [unwired: 8 in, 2 out]
        n64 = call <vilib>:"Check if File or Folder Exists.vi"("path"=w363) -> ("file or folder exists?"=w348:bool)  [unwired: 8 in, 2 out]
        n65 = Select(t=w344, s=w346, f=w345) -> (s? t:f=w343:T40[])
        n66 = Compound Arithmetic op=AND(w351, w349, w348, w347) -> (w340:bool)
        n67 = case shown="False" w340 {
          tunnel: [ENUM_ACT_State."Configuring" ("State") ENUM_ACT_State."Stopping" ("State")] -> w361
          tunnel: [w370 w387] -> w342
          tunnel: w351 -> [w383 _]
          tunnel: w349 -> [w379 _]
          tunnel: w348 -> [w377 _]
          tunnel: w347 -> [w372 _]
          tunnel: w343 -> [w365 w386]
          frame False {
            w374 = T40[] [enum."Config HW Drive Get", enum."Config HW Drive Save"] items=["No Action", "Reset Time", "Reset All", "Open HW References", "Control FX Stop", "Control FX Mode 1", "Control FX Mode 2", "Set Robot Start Position", "Config HW Steer Set", "Config HW Steer Get", "Config HW Steer Save", "Config HW Steer Read", "Config HW Drive Set", "Config HW Drive Get", "Config HW Drive Save", "Config HW Drive Read", "Config HW Specific Set", "Config HW Specific Get", "Config HW Specific Save", "Config HW Specific Read", "Config System Save", "Config System Read", "Config From FP", "Start HW Steer Set", "Default HW Steer Set", "Defalut HW Drive Set"] ("Action")
            w373 = T40[] [] items=["No Action", "Reset Time", "Reset All", "Open HW References", "Control FX Stop", "Control FX Mode 1", "Control FX Mode 2", "Set Robot Start Position", "Config HW Steer Set", "Config HW Steer Get", "Config HW Steer Save", "Config HW Steer Read", "Config HW Drive Set", "Config HW Drive Get", "Config HW Drive Save", "Config HW Drive Read", "Config HW Specific Set", "Config HW Specific Get", "Config HW Specific Save", "Config HW Specific Read", "Config System Save", "Config System Read", "Config From FP", "Start HW Steer Set", "Default HW Steer Set", "Defalut HW Drive Set"] ("Action")
            w375 = T40[] [enum."Config HW Steer Get", enum."Config HW Steer Save"] items=["No Action", "Reset Time", "Reset All", "Open HW References", "Control FX Stop", "Control FX Mode 1", "Control FX Mode 2", "Set Robot Start Position", "Config HW Steer Set", "Config HW Steer Get", "Config HW Steer Save", "Config HW Steer Read", "Config HW Drive Set", "Config HW Drive Get", "Config HW Drive Save", "Config HW Drive Read", "Config HW Specific Set", "Config HW Specific Get", "Config HW Specific Save", "Config HW Specific Read", "Config System Save", "Config System Read", "Config From FP", "Start HW Steer Set", "Default HW Steer Set", "Defalut HW Drive Set"] ("Action")
            w376 = T40[] [] items=["No Action", "Reset Time", "Reset All", "Open HW References", "Control FX Stop", "Control FX Mode 1", "Control FX Mode 2", "Set Robot Start Position", "Config HW Steer Set", "Config HW Steer Get", "Config HW Steer Save", "Config HW Steer Read", "Config HW Drive Set", "Config HW Drive Get", "Config HW Drive Save", "Config HW Drive Read", "Config HW Specific Set", "Config HW Specific Get", "Config HW Specific Save", "Config HW Specific Read", "Config System Save", "Config System Read", "Config From FP", "Start HW Steer Set", "Default HW Steer Set", "Defalut HW Drive Set"] ("Action")
            # "Config Files Missing"
            n68 = Select(t=w376, s=w377, f=w375) -> (s? t:f=w366:T40[])
            n69 = Select(t=ENUM_ACT_Action."No Action" ("Action"), s=w379, f=ENUM_ACT_Action."Config System Save" ("Action")) -> (s? t:f=w368:T40)
            n70 = Select(t=ENUM_ACT_Action."No Action" ("Action"), s=w383, f=ENUM_ACT_Action."Config HW Specific Save" ("Action")) -> (s? t:f=w367:T40)
            n71 = Select(t=w373, s=w372, f=w374) -> (s? t:f=w369:T40[])
            n72 = Build Array (concatenate)(w367, w368, w365, w366, w369) -> (w370:T40[])
          }
          frame True {
            w385 = T40[] [enum."Config HW Specific Read", enum."Config System Read", enum."Config HW Drive Read", enum."Config HW Steer Read"] items=["No Action", "Reset Time", "Reset All", "Open HW References", "Control FX Stop", "Control FX Mode 1", "Control FX Mode 2", "Set Robot Start Position", "Config HW Steer Set", "Config HW Steer Get", "Config HW Steer Save", "Config HW Steer Read", "Config HW Drive Set", "Config HW Drive Get", "Config HW Drive Save", "Config HW Drive Read", "Config HW Specific Set", "Config HW Specific Get", "Config HW Specific Save", "Config HW Specific Read", "Config System Save", "Config System Read", "Config From FP", "Start HW Steer Set", "Default HW Steer Set", "Defalut HW Drive Set"] ("Actions")
            w384 = T40[] [enum."Default HW Steer Set", enum."Defalut HW Drive Set", enum."Config HW Steer Set", enum."Config HW Specific Set", enum."Config HW Drive Set", enum."Start HW Steer Set"] items=["No Action", "Reset Time", "Reset All", "Open HW References", "Control FX Stop", "Control FX Mode 1", "Control FX Mode 2", "Set Robot Start Position", "Config HW Steer Set", "Config HW Steer Get", "Config HW Steer Save", "Config HW Steer Read", "Config HW Drive Set", "Config HW Drive Get", "Config HW Drive Save", "Config HW Drive Read", "Config HW Specific Set", "Config HW Specific Get", "Config HW Specific Save", "Config HW Specific Read", "Config System Save", "Config System Read", "Config From FP", "Start HW Steer Set", "Default HW Steer Set", "Defalut HW Drive Set"] ("Actions")
            # "All Config File are present"
            n73 = Build Array (concatenate)(w385, w386, w384) -> (w387:T40[])
          }
        }
      }
      frame "Stopping" {
        (unwired) TRUE
        w390 = T40[] [enum."Control FX Stop"] items=["No Action", "Reset Time", "Reset All", "Open HW References", "Control FX Stop", "Control FX Mode 1", "Control FX Mode 2", "Set Robot Start Position", "Config HW Steer Set", "Config HW Steer Get", "Config HW Steer Save", "Config HW Steer Read", "Config HW Drive Set", "Config HW Drive Get", "Config HW Drive Save", "Config HW Drive Read", "Config HW Specific Set", "Config HW Specific Get", "Config HW Specific Save", "Config HW Specific Read", "Config System Save", "Config System Read", "Config From FP", "Start HW Steer Set", "Default HW Steer Set", "Defalut HW Drive Set"] ("Actions")
        n74 = Unbundle By Name(w393) -> ("ACT Input.Mode"=w394:T29)
        n75 = case shown="\"STOP\"" w394 {
          tunnel: w393 -> [w397 w400 w403 w406 w409]
          tunnel: [w397 w400 w403 w406 w409] -> w392
          tunnel: [ENUM_ACT_State."Stopping" ("State") ENUM_ACT_State."Moving Mode 1" ("State") ENUM_ACT_State."Moving Mode 2" ("State") ENUM_ACT_State."Moving Mode 2" ("State") ENUM_ACT_State."Moving Mode 2" ("State")] -> w391
          tunnel: [w395 w398 w401 w404 w407] -> w389
          tunnel: w390 -> [w395 w398 w401 w404 w407]
          frame "STOP" {
          }
          frame "Move" {
          }
          frame "Turret Manual" {
          }
          frame "Trans Manual Angle Auto" {
          }
          frame "Turret Auto Angle" {
          }
        }
      }
      frame "Initializing HW" {
        (unwired) TRUE
        w411 = T40[] [enum."Control FX Stop"] items=["No Action", "Reset Time", "Reset All", "Open HW References", "Control FX Stop", "Control FX Mode 1", "Control FX Mode 2", "Set Robot Start Position", "Config HW Steer Set", "Config HW Steer Get", "Config HW Steer Save", "Config HW Steer Read", "Config HW Drive Set", "Config HW Drive Get", "Config HW Drive Save", "Config HW Drive Read", "Config HW Specific Set", "Config HW Specific Get", "Config HW Specific Save", "Config HW Specific Read", "Config System Save", "Config System Read", "Config From FP", "Start HW Steer Set", "Default HW Steer Set", "Defalut HW Drive Set"] ("Actions")
        n76 = Unbundle By Name(w414) -> ("ACT Input.Mode"=w415:T29)
        n77 = case shown="\"Trans Manual Angle Auto\"" w415 {
          tunnel: w414 -> [w418 w421 w424 w427 w430]
          tunnel: [w418 w421 w424 w427 w430] -> w413
          tunnel: [ENUM_ACT_State."Stopping" ("State") ENUM_ACT_State."Moving Mode 1" ("State") ENUM_ACT_State."Moving Mode 2" ("State") ENUM_ACT_State."Moving Mode 2" ("State") ENUM_ACT_State."Moving Mode 2" ("State")] -> w412
          tunnel: [w416 w419 w422 w425 w428] -> w410
          tunnel: w411 -> [w416 w419 w422 w425 w428]
          frame "STOP" {
          }
          frame "Move" {
          }
          frame "Turret Manual" {
          }
          frame "Trans Manual Angle Auto" {
          }
          frame "Turret Auto Angle" {
          }
        }
      }
      frame "Moving Mode 1" {
        w431 = T40[] [enum."Control FX Stop"] items=["No Action", "Reset Time", "Reset All", "Open HW References", "Control FX Stop", "Control FX Mode 1", "Control FX Mode 2", "Set Robot Start Position", "Config HW Steer Set", "Config HW Steer Get", "Config HW Steer Save", "Config HW Steer Read", "Config HW Drive Set", "Config HW Drive Get", "Config HW Drive Save", "Config HW Drive Read", "Config HW Specific Set", "Config HW Specific Get", "Config HW Specific Save", "Config HW Specific Read", "Config System Save", "Config System Read", "Config From FP", "Start HW Steer Set", "Default HW Steer Set", "Defalut HW Drive Set"] ("Actions")
        n78 = Unbundle By Name(w434) -> ("ACT Input.Mode"=w436:T29)
        n79 = case shown="\"Turret Auto Angle\"" w436 {
          tunnel: [ENUM_ACT_State."Stopping" ("State") ENUM_ACT_State."Moving Mode 2" ("State") ENUM_ACT_State."Moving Mode 2" ("State") ENUM_ACT_State."Moving Mode 2" ("State") w451] -> w437
          tunnel: w434 -> [w440 w443 w446 w449 w452]
          tunnel: [w440 w443 w446 w449 w452] -> w435
          tunnel: w433 -> [_ _ _ _ w451]
          tunnel: [w438 w441 w444 w447 w450] -> w432
          tunnel: w431 -> [w438 w441 w444 w447 _]
          frame "STOP" {
          }
          frame "Turret Manual" {
          }
          frame "Trans Manual Angle Auto" {
          }
          frame "Turret Auto Angle" {
          }
          frame "Move" {
            w450 = T40[] [enum."Control FX Mode 1"] items=["No Action", "Reset Time", "Reset All", "Open HW References", "Control FX Stop", "Control FX Mode 1", "Control FX Mode 2", "Set Robot Start Position", "Config HW Steer Set", "Config HW Steer Get", "Config HW Steer Save", "Config HW Steer Read", "Config HW Drive Set", "Config HW Drive Get", "Config HW Drive Save", "Config HW Drive Read", "Config HW Specific Set", "Config HW Specific Get", "Config HW Specific Save", "Config HW Specific Read", "Config System Save", "Config System Read", "Config From FP", "Start HW Steer Set", "Default HW Steer Set", "Defalut HW Drive Set"] ("Actions")
          }
        }
      }
      frame "Moving Mode 2" {
        w454 = T40[] [enum."Control FX Stop"] items=["No Action", "Reset Time", "Reset All", "Open HW References", "Control FX Stop", "Control FX Mode 1", "Control FX Mode 2", "Set Robot Start Position", "Config HW Steer Set", "Config HW Steer Get", "Config HW Steer Save", "Config HW Steer Read", "Config HW Drive Set", "Config HW Drive Get", "Config HW Drive Save", "Config HW Drive Read", "Config HW Specific Set", "Config HW Specific Get", "Config HW Specific Save", "Config HW Specific Read", "Config System Save", "Config System Read", "Config From FP", "Start HW Steer Set", "Default HW Steer Set", "Defalut HW Drive Set"] ("Actions")
        n80 = Unbundle By Name(w456) -> ("ACT Input.Mode"=w458:T29)
        n81 = case shown="\"Turret Auto Angle\"" w458 {
          tunnel: [ENUM_ACT_State."Stopping" ("State") w463 w466 w469 ENUM_ACT_State."Moving Mode 1" ("State")] -> w459
          tunnel: w456 -> [w462 w465 w468 w471 w474]
          tunnel: [w462 w465 w468 w471 w474] -> w457
          tunnel: w455 -> [_ w463 w466 w469 _]
          tunnel: [w460 w464 w467 w470 w472] -> w453
          tunnel: w454 -> [w460 _ _ _ w472]
          frame "STOP" {
          }
          frame "Turret Manual" {
            w464 = T40[] [enum."Control FX Mode 2"] items=["No Action", "Reset Time", "Reset All", "Open HW References", "Control FX Stop", "Control FX Mode 1", "Control FX Mode 2", "Set Robot Start Position", "Config HW Steer Set", "Config HW Steer Get", "Config HW Steer Save", "Config HW Steer Read", "Config HW Drive Set", "Config HW Drive Get", "Config HW Drive Save", "Config HW Drive Read", "Config HW Specific Set", "Config HW Specific Get", "Config HW Specific Save", "Config HW Specific Read", "Config System Save", "Config System Read", "Config From FP", "Start HW Steer Set", "Default HW Steer Set", "Defalut HW Drive Set"] ("Actions")
          }
          frame "Trans Manual Angle Auto" {
            w467 = T40[] [enum."Control FX Mode 2"] items=["No Action", "Reset Time", "Reset All", "Open HW References", "Control FX Stop", "Control FX Mode 1", "Control FX Mode 2", "Set Robot Start Position", "Config HW Steer Set", "Config HW Steer Get", "Config HW Steer Save", "Config HW Steer Read", "Config HW Drive Set", "Config HW Drive Get", "Config HW Drive Save", "Config HW Drive Read", "Config HW Specific Set", "Config HW Specific Get", "Config HW Specific Save", "Config HW Specific Read", "Config System Save", "Config System Read", "Config From FP", "Start HW Steer Set", "Default HW Steer Set", "Defalut HW Drive Set"] ("Actions")
          }
          frame "Turret Auto Angle" {
            w470 = T40[] [enum."Control FX Mode 2"] items=["No Action", "Reset Time", "Reset All", "Open HW References", "Control FX Stop", "Control FX Mode 1", "Control FX Mode 2", "Set Robot Start Position", "Config HW Steer Set", "Config HW Steer Get", "Config HW Steer Save", "Config HW Steer Read", "Config HW Drive Set", "Config HW Drive Get", "Config HW Drive Save", "Config HW Drive Read", "Config HW Specific Set", "Config HW Specific Get", "Config HW Specific Save", "Config HW Specific Read", "Config System Save", "Config System Read", "Config From FP", "Start HW Steer Set", "Default HW Steer Set", "Defalut HW Drive Set"] ("Actions")
          }
          frame "Move" {
          }
        }
      }
      frame "Shutdown" {
        w475 = T40[] [enum."Reset All"] items=["No Action", "Reset Time", "Reset All", "Open HW References", "Control FX Stop", "Control FX Mode 1", "Control FX Mode 2", "Set Robot Start Position", "Config HW Steer Set", "Config HW Steer Get", "Config HW Steer Save", "Config HW Steer Read", "Config HW Drive Set", "Config HW Drive Get", "Config HW Drive Save", "Config HW Drive Read", "Config HW Specific Set", "Config HW Specific Get", "Config HW Specific Save", "Config HW Specific Read", "Config System Save", "Config System Read", "Config From FP", "Start HW Steer Set", "Default HW Steer Set", "Defalut HW Drive Set"] ("Actions")
      }
    }
    n82 = case shown="True" w77 {
      tunnel: w76 -> [_ w480]
      tunnel: [_ w478] -> w75
      frame False {
      }
      frame True {
        # "Change Detected"
        n83 = call "Search Unsorted 1D Array.vim"("element"=TRUE, "unsorted 1D array"=w480) -> ("index of element"=w479:i32)  [unwired: 9 in]
        n84 = case shown="1" w479 {
          tunnel: [w482 w483 w484 w485 w486 w487 w488] -> w478
          frame ..0 {
            w482 = T40[] [enum."Config HW Specific Read", enum."Config HW Steer Read", enum."Config HW Drive Read", enum."Config System Read"] items=["No Action", "Reset Time", "Reset All", "Open HW References", "Control FX Stop", "Control FX Mode 1", "Control FX Mode 2", "Set Robot Start Position", "Config HW Steer Set", "Config HW Steer Get", "Config HW Steer Save", "Config HW Steer Read", "Config HW Drive Set", "Config HW Drive Get", "Config HW Drive Save", "Config HW Drive Read", "Config HW Specific Set", "Config HW Specific Get", "Config HW Specific Save", "Config HW Specific Read", "Config System Save", "Config System Read", "Config From FP", "Start HW Steer Set", "Default HW Steer Set", "Defalut HW Drive Set"] ("Actions")
            # "Read Config"
          }
          frame 1 {
            w483 = T40[] [enum."Config From FP"] items=["No Action", "Reset Time", "Reset All", "Open HW References", "Control FX Stop", "Control FX Mode 1", "Control FX Mode 2", "Set Robot Start Position", "Config HW Steer Set", "Config HW Steer Get", "Config HW Steer Save", "Config HW Steer Read", "Config HW Drive Set", "Config HW Drive Get", "Config HW Drive Save", "Config HW Drive Read", "Config HW Specific Set", "Config HW Specific Get", "Config HW Specific Save", "Config HW Specific Read", "Config System Save", "Config System Read", "Config From FP", "Start HW Steer Set", "Default HW Steer Set", "Defalut HW Drive Set"] ("Actions")
            # "Updated Config"
          }
          frame 2 {
            w484 = T40[] [enum."Config HW Steer Set", enum."Config HW Steer Save"] items=["No Action", "Reset Time", "Reset All", "Open HW References", "Control FX Stop", "Control FX Mode 1", "Control FX Mode 2", "Set Robot Start Position", "Config HW Steer Set", "Config HW Steer Get", "Config HW Steer Save", "Config HW Steer Read", "Config HW Drive Set", "Config HW Drive Get", "Config HW Drive Save", "Config HW Drive Read", "Config HW Specific Set", "Config HW Specific Get", "Config HW Specific Save", "Config HW Specific Read", "Config System Save", "Config System Read", "Config From FP", "Start HW Steer Set", "Default HW Steer Set", "Defalut HW Drive Set"] ("Actions")
            # "Steer Change"
          }
          frame 3 {
            w485 = T40[] [enum."Config HW Drive Set", enum."Config HW Drive Save"] items=["No Action", "Reset Time", "Reset All", "Open HW References", "Control FX Stop", "Control FX Mode 1", "Control FX Mode 2", "Set Robot Start Position", "Config HW Steer Set", "Config HW Steer Get", "Config HW Steer Save", "Config HW Steer Read", "Config HW Drive Set", "Config HW Drive Get", "Config HW Drive Save", "Config HW Drive Read", "Config HW Specific Set", "Config HW Specific Get", "Config HW Specific Save", "Config HW Specific Read", "Config System Save", "Config System Read", "Config From FP", "Start HW Steer Set", "Default HW Steer Set", "Defalut HW Drive Set"] ("Actions")
            # "Drive Change"
          }
          frame 4 {
            w486 = T40[] [enum."Config HW Specific Save"] items=["No Action", "Reset Time", "Reset All", "Open HW References", "Control FX Stop", "Control FX Mode 1", "Control FX Mode 2", "Set Robot Start Position", "Config HW Steer Set", "Config HW Steer Get", "Config HW Steer Save", "Config HW Steer Read", "Config HW Drive Set", "Config HW Drive Get", "Config HW Drive Save", "Config HW Drive Read", "Config HW Specific Set", "Config HW Specific Get", "Config HW Specific Save", "Config HW Specific Read", "Config System Save", "Config System Read", "Config From FP", "Start HW Steer Set", "Default HW Steer Set", "Defalut HW Drive Set"] ("Actions")
            # "Specific Change"
          }
          frame 5 {
            w487 = T40[] [enum."Config System Save"] items=["No Action", "Reset Time", "Reset All", "Open HW References", "Control FX Stop", "Control FX Mode 1", "Control FX Mode 2", "Set Robot Start Position", "Config HW Steer Set", "Config HW Steer Get", "Config HW Steer Save", "Config HW Steer Read", "Config HW Drive Set", "Config HW Drive Get", "Config HW Drive Save", "Config HW Drive Read", "Config HW Specific Set", "Config HW Specific Get", "Config HW Specific Save", "Config HW Specific Read", "Config System Save", "Config System Read", "Config From FP", "Start HW Steer Set", "Default HW Steer Set", "Defalut HW Drive Set"] ("Actions")
            # "System Change"
          }
          frame 6.. {
            w488 = T40[] [enum."Config HW Specific Get"] items=["No Action", "Reset Time", "Reset All", "Open HW References", "Control FX Stop", "Control FX Mode 1", "Control FX Mode 2", "Set Robot Start Position", "Config HW Steer Set", "Config HW Steer Get", "Config HW Steer Save", "Config HW Steer Read", "Config HW Drive Set", "Config HW Drive Get", "Config HW Drive Save", "Config HW Drive Read", "Config HW Specific Set", "Config HW Specific Get", "Config HW Specific Save", "Config HW Specific Read", "Config System Save", "Config System Read", "Config From FP", "Start HW Steer Set", "Default HW Steer Set", "Defalut HW Drive Set"] ("Actions")
            # "System Change"
          }
        }
      }
    }
    n85 = global write "Global_ACT_Data Out.vi" "ACT_Template_STATE"(w65) -> ()
    n86 = Bundle By Name(cluster=w105, "Previous State"=w65, "State"=w104) -> (w106:T39)
    n87 = Build Array (concatenate)(w94, w75) -> (w90:T40[])
    n88 = for {
      tunnel: w90 -> [w139] mode=indexing
      shift-right: [w138] -> w89
      shift-left: w106 -> [w137]
      n89 = case shown="\"Config HW Steer Save\"" w139 {
        tunnel: w137 -> [w140 w143 w144 w149 w156 w157 w158 w159 w161 w175 w189 w197 w200 w213 w227 w235 w241 w252 w264 w271 w278 w285 w298 w316 w318 w325]
        tunnel: [w140 w142 w144 w150 w156 w157 w158 w159 w160 w174 w190 w198 w199 w212 w228 w236 w243 w254 w265 w272 w279 w286 w299 w316 w317 w324] -> w138
        frame "No Action" {
        }
        frame "Reset Time" {
          n90 = Unbundle By Name(w143) -> ("Current Time"=w141:timestamp)
          n91 = Bundle By Name(cluster=w143, "Start Time"=w141) -> (w142:T39)
        }
        frame "Reset All" {
        }
        frame "Open HW References" {
          n92 = Unbundle By Name(w149) -> ("Config Specific.Specific Data"=w148:T15[])
          n93 = for {
            tunnel: w148 -> [w155] mode=indexing
            tunnel: [w153] -> w147 mode=indexing
            tunnel: [w154] -> w146 mode=indexing
            tunnel: [w152] -> _
            tunnel: [w151] -> _
            n94 = call "Open HW References.vi"("Module Azimuth Config Data"=w155) -> (0:"Error Out"=w152:errorcluster, 1:"Error Out"=w151:errorcluster, "Module Drive Ref Out"=w154:T32, "Module Steer Ref Out"=w153:T32)  [unwired: 7 in]
          }
          n95 = Bundle By Name(cluster=w149, "Steer Refs"=w147, "Drive Refs"=w146, "HW OPEN"=TRUE) -> (w150:T39)
        }
        frame "Control FX Stop" {
          # "#Fix"
        }
        frame "Control FX Mode 1" {
          # "#Fix"
        }
        frame "Control FX Mode 2" {
          # "#Fix"
        }
        frame "Set Robot Start Position" {
          # "#Fix"
        }
        frame "Config HW Steer Set" {
          n96 = in-place {
            n97 = in-place-cluster #1(w161) -> ("Config Steer"=w164:T8, "Steer Refs"=w166:T32[])  [unwired: 1 out]
            n98 = for {
              tunnel: w166 -> [w173] mode=indexing
              tunnel: [w172] -> w165 mode=indexing
              shift-right: [w170] -> w163
              shift-left: w164 -> [w171]
              n99 = call "Config Steer Module Get-Set.vi"("Start With Default"=FALSE, "Get(f) Set(t)"=TRUE, "Set Steer Values"=w171, "Send Cmd Timout(ms)"=u32 300, "Steer Refs"=w173) -> ("Steer Refs Out"=w172:T32, "Steer Config Out"=w170:T8)  [unwired: 3 in, 2 out]
            }
            n100 = in-place-cluster #1("Config Steer"=w163, "Steer Refs"=w165, "Steer Change"=FALSE ("Update Display")) -> (w160:T39)
          }
        }
        frame "Config HW Steer Get" {
          n101 = in-place {
            n102 = in-place-cluster #2(w175) -> ("Config Steer"=w183:T8, "Steer Refs"=w177:T32[])  [unwired: 1 out]
            n103 = Index Array(array=w177) -> (element=w178:T32)  [unwired: 1 in]
            n104 = call "Config Steer Module Get-Set.vi"("Start With Default"=FALSE, "Get(f) Set(t)"=FALSE, "Set Steer Values"=w183, "Send Cmd Timout(ms)"=u32 300, "Steer Refs"=w178) -> ("Steer Config Out"=w182:T8)  [unwired: 3 in, 3 out]
            n105 = in-place-cluster #2("Config Steer"=w182, "Steer Refs"=w177, "Update Display"=TRUE) -> (w174:T39)
          }
        }
        frame "Config HW Steer Save" {
          n106 = Unbundle By Name(w189) -> ("Team Folder"=w187:path, "Config Steer"=w184:T8)
          n107 = call "RWA_File Config.vim"("Read(f) Save(t)"=TRUE ("Read(f) Write(t)"), "Target Folder Folder"=w187, "Any Config"=w184) -> ("Any Config Out"=w188:T8)  [unwired: 4 in, 4 out]
          n108 = Bundle By Name(cluster=w189, "Config Steer"=w188, "Steer Change"=FALSE) -> (w190:T39)
        }
        frame "Config HW Steer Read" {
          n109 = Unbundle By Name(w197) -> ("Team Folder"=w191:path, "Config Steer"=w192:T8)
          n110 = call "RWA_File Config.vim"("Read(f) Save(t)"=FALSE ("Read(f) Write(t)"), "Target Folder Folder"=w191, "Any Config"=w192) -> ("Any Config Out"=w194:T8)  [unwired: 4 in, 4 out]
          n111 = Not Equal?(x=w192, y=w194) -> (x != y?=w193:bool)
          n112 = Bundle By Name(cluster=w197, "Steer Change"=w193, "Config Steer"=w194, "Update Display"=TRUE) -> (w198:T39)
        }
        frame "Config HW Drive Set" {
          n113 = in-place {
            n114 = in-place-cluster #3(w200) -> ("Config Drive"=w203:T1, "Drive Refs"=w205:T32[])  [unwired: 1 out]
            n115 = for {
              tunnel: w205 -> [w211] mode=indexing
              tunnel: [w210] -> w204 mode=indexing
              shift-right: [w208] -> w202
              shift-left: w203 -> [w209]
              n116 = call "Config Drive Module Get-Set.vi"("Start with Default"=FALSE ("Start With Default"), "Get(f) Set(t)"=TRUE, "Set Drive Config"=w209, "Drive Refs"=w211) -> ("Drive Refs Out"=w210:T32, "Drive Config Out"=w208:T1)  [unwired: 5 in, 1 out]
            }
            n117 = in-place-cluster #3("Config Drive"=w202, "Drive Refs"=w204, "Drive Change"=FALSE) -> (w199:T39)
          }
        }
        frame "Config HW Drive Get" {
          n118 = in-place {
            n119 = in-place-cluster #4(w213) -> ("Config Drive"=w221:T1, "Drive Refs"=w216:T32[])  [unwired: 1 out]
            n120 = Index Array(array=w216, index=3) -> (element=w217:T32)
            n121 = call "Config Drive Module Get-Set.vi"("Start with Default"=FALSE ("Start With Default"), "Get(f) Set(t)"=FALSE, "Set Drive Config"=w221, "Drive Refs"=w217) -> ("Drive Config Out"=w220:T1)  [unwired: 5 in, 2 out]
            n122 = in-place-cluster #4("Config Drive"=w220, "Drive Refs"=w216, "Update Display"=TRUE) -> (w212:T39)
          }
        }
        frame "Config HW Drive Save" {
          n123 = Unbundle By Name(w227) -> ("Team Folder"=w224:path, "Config Drive"=w226:T1)
          n124 = call "RWA_File Config.vim"("Read(f) Save(t)"=TRUE ("Read(f) Write(t)"), "Target Folder Folder"=w224, "Any Config"=w226) -> ("Any Config Out"=w225:T1)  [unwired: 4 in, 4 out]
          n125 = Bundle By Name(cluster=w227, "Config Drive"=w225, "Drive Change"=FALSE) -> (w228:T39)
        }
        frame "Config HW Drive Read" {
          n126 = Unbundle By Name(w235) -> ("Team Folder"=w234:path, "Config Drive"=w230:T1)
          n127 = call "RWA_File Config.vim"("Read(f) Save(t)"=FALSE ("Read(f) Write(t)"), "Target Folder Folder"=w234, "Any Config"=w230) -> ("Any Config Out"=w231:T1)  [unwired: 4 in, 4 out]
          n128 = Not Equal?(x=w230, y=w231) -> (x != y?=w229:bool)
          n129 = Bundle By Name(cluster=w235, "Drive Change"=w229, "Config Drive"=w231, "Update Display"=TRUE) -> (w236:T39)
        }
        frame "Config HW Specific Set" {
          n130 = Unbundle By Name(w241) -> ("Config Specific.Specific Data"=w239:T15[], "HW Out.Swerve Read"=w240:T25)
          n131 = Cluster To Array(cluster=w240) -> (array=w237:T26[])
          n132 = for {
            tunnel: w239 -> [w246] mode=indexing
            tunnel: [w247] -> w238 mode=indexing
            tunnel: w237 -> [w245] mode=indexing
            n133 = Unbundle By Name(w245) -> ("Angle"=w244:T24)
            n134 = Bundle By Name(cluster=w246, "Encoder Start Value"=w244) -> (w247:T15)
          }
          n135 = Bundle By Name(cluster=w241, "Config Specific.Specific Data"=w238, "Specific Change"=TRUE) -> (w243:T39)
        }
        frame "Config HW Specific Get" {
          n136 = Unbundle By Name(w252) -> ("Config Specific.Specific Data"=w250:T15[], "HW Out.Swerve Read"=w251:T25)
          n137 = Cluster To Array(cluster=w251) -> (array=w248:T26[])
          n138 = for {
            tunnel: w250 -> [w257] mode=indexing
            tunnel: [w258] -> w249 mode=indexing
            tunnel: w248 -> [w256] mode=indexing
            n139 = Unbundle By Name(w256) -> ("Angle"=w255:T24)
            n140 = Bundle By Name(cluster=w257, "Encoder Start Value"=w255) -> (w258:T15)
          }
          n141 = Bundle By Name(cluster=w252, "Config Specific.Specific Data"=w249, "Specific Change"=TRUE) -> (w254:T39)
        }
        frame "Config HW Specific Save" {
          n142 = Unbundle By Name(w264) -> ("Team Folder"=w263:path, "Config Specific"=w260:T14)
          n143 = call "RWA_File Config.vim"("Read(f) Save(t)"=TRUE ("Read(f) Write(t)"), "Target Folder Folder"=w263, "Any Config"=w260) -> ("Any Config Out"=w259:T14)  [unwired: 4 in, 4 out]
          n144 = Bundle By Name(cluster=w264, "Config Specific"=w259, "Specific Change"=FALSE) -> (w265:T39)
        }
        frame "Config HW Specific Read" {
          n145 = Unbundle By Name(w271) -> ("Team Folder"=w268:path, "Config System"=w270:T17)
          n146 = call "RWA_File Config.vim"("Read(f) Save(t)"=FALSE ("Read(f) Write(t)"), "Target Folder Folder"=w268, "Any Config"=w270) -> ("Any Config Out"=w269:T17)  [unwired: 4 in, 4 out]
          n147 = Bundle By Name(cluster=w271, "Config System"=w269, "Update Display"=TRUE) -> (w272:T39)
        }
        frame "Config System Save" {
          n148 = Unbundle By Name(w278) -> ("Team Folder"=w275:path, "Config System"=w277:T17)
          n149 = call "RWA_File Config.vim"("Read(f) Save(t)"=TRUE ("Read(f) Write(t)"), "Target Folder Folder"=w275, "Any Config"=w277) -> ("Any Config Out"=w276:T17)  [unwired: 4 in, 4 out]
          n150 = Bundle By Name(cluster=w278, "Config System"=w276, "System Change"=FALSE) -> (w279:T39)
        }
        frame "Config System Read" {
          n151 = Unbundle By Name(w285) -> ("Team Folder"=w282:path, "Config System"=w284:T17)
          n152 = call "RWA_File Config.vim"("Read(f) Save(t)"=FALSE ("Read(f) Write(t)"), "Target Folder Folder"=w282, "Any Config"=w284) -> ("Any Config Out"=w283:T17)  [unwired: 4 in, 4 out]
          n153 = Bundle By Name(cluster=w285, "Config System"=w283, "Update Display"=TRUE) -> (w286:T39)
        }
        frame "Config From FP" {
          n154 = Unbundle By Name(w298) -> ("Current Time"=w315:timestamp)
          n155 = Unbundle By Name(w298) -> ("Config Drive"=w304:T1, "Config Drive.Drive HW Ver"=w302:u64, "Config Steer"=w303:T8, "Config Steer.Steer HW Ver"=w300:u64)
          n156 = Unbundle By Name(w298) -> ("Config Specific"=w309:T14, "Config Specific.Specific HW Ver"=w308:u64)
          n157 = Unbundle By Name(w298) -> ("Config System"=w310:T17, "Config System.System Ver"=w312:u64)
          n158 = call "Date Stamp.vi"("Time"=w315) -> ("U64 Out"=w301:u64)  [unwired: 5 in, 1 out]
          n159 = Not Equal?(x=w310, y="Config System") -> (x != y?=w290:bool)
          n160 = Not Equal?(x="Config Specific", y=w309) -> (x != y?=w287:bool)
          n161 = Select(t=w301, s=w290, f=w312) -> (s? t:f=w311:u64)
          n162 = Select(t=w301, s=w287, f=w308) -> (s? t:f=w306:u64)
          n163 = Not Equal?(x="Config Steer", y=w303) -> (x != y?=w288:bool)
          n164 = Bundle By Name(cluster="Config System", "System Ver"=w311) -> (w314:T17)
          n165 = Not Equal?(x="Config Drive", y=w304) -> (x != y?=w291:bool)
          n166 = Select(t=w301, s=w288, f=w300) -> (s? t:f=w292:u64)
          n167 = Bundle By Name(cluster="Config Steer", "Steer HW Ver"=w292) -> (w293:T8)
          n168 = Bundle By Name(cluster="Config Specific", "Specific HW Ver"=w306) -> (w305:T14)
          n169 = Select(t=w301, s=w291, f=w302) -> (s? t:f=w296:u64)
          n170 = Bundle By Name(cluster="Config Drive", "Drive HW Ver"=w296) -> (w295:T1)
          n171 = Bundle By Name(cluster=w298, "Config Drive"=w295, "Drive Change"=w291, "Config Steer"=w293, "Steer Change"=w288, "Config System"=w314, "System Change"=w290, "Config Specific"=w305, "Specific Change"=w287, "Update Display"=TRUE) -> (w299:T39)
        }
        frame "Start HW Steer Set" {
        }
        frame "Default HW Steer Set" {
          n172 = in-place {
            w319 = TRUE ("Drive Change")
            n173 = in-place-cluster #5(w318) -> ("Steer Refs"=w321:T32[])  [unwired: 2 out]
            n174 = for {
              tunnel: w321 -> [w323] mode=indexing
              tunnel: [w322] -> w320 mode=indexing
              n175 = call <vilib>:"CTRE_Phoenix_MotorControl_FactoryDefault.vi"("PhoenixMotorControlDevRef"=w323) -> ("PhoenixMotorControlDevRef"=w322:T32)  [unwired: 9 in, 1 out]
            }
            n176 = in-place-cluster #5("Steer Refs"=w320, "Steer Change"=w319, "Specific Change"=w319) -> (w317:T39)
          }
        }
        frame "Defalut HW Drive Set" {
          n177 = in-place {
            n178 = in-place-cluster #6(w325) -> ("Drive Refs"=w328:T32[])  [unwired: 1 out]
            n179 = for {
              tunnel: w328 -> [w330] mode=indexing
              tunnel: [w329] -> w327 mode=indexing
              n180 = call <vilib>:"SPARK Restore Factory Default.vi"("MotorControlDeviceRef"=w330) -> ("MotorControlDeviceRef"=w329:T32)  [unwired: 9 in, 1 out]
            }
            n181 = in-place-cluster #6("Drive Refs"=w327, "Drive Change"=TRUE) -> (w324:T39)
          }
        }
      }
    }
    n182 = Unbundle By Name(w89) -> ("Config System"=w45:T17, "Config Drive"=w46:T1, "Config Steer"=w86:T8, "Update Display"=w87:bool, "Config System"=w69:T17, "Config Specific"=w53:T14)
    n183 = Unbundle By Name(w89) -> ("State"=w85:T38)
    n184 = Unbundle By Name(w89) -> ("Cycle Time(S)"=w91:dbl)
    "Cycle Time (S)" <- w91
    n185 = Unbundle By Name(w89) -> ("ACT Input"=→"CMD":T28, "HW Out"=w83:T23, "System Output"=w74:T22)
    "HW Output" <- w83
    "System Config" <- w74
    n186 = case shown="\"Startup\", \"Configuring\"" w85 {
      frame "Startup", "Configuring" {
        # "#Fix"
      }
      frame Default {
      }
    }
    n187 = case shown="False" w87 {
      tunnel: w86 -> [_ w491]
      tunnel: w69 -> [_ w493]
      tunnel: w53 -> [_ w492]
      tunnel: w46 -> [_ w490]
      tunnel: w45 -> [_ w489]
      frame False {
      }
      frame True {
        n188 = local write "Config System"(w493) -> ()
        n189 = local write "Config Specific"(w492) -> ()
        n190 = local write "Config Steer"(w491) -> ()
        n191 = local write "Config System"(w489) -> ()
        n192 = local write "Config Drive"(w490) -> ()
      }
    }
    n193 = global write "Global_ACT_Data Out.vi" "ACT_Template_System Output"(w74) -> ()
    n194 = global write "Global_ACT_Data Out.vi" "ACT_Template_HW Output"(w83) -> ()
    n195 = global write "Global_ACT_Data Out.vi" "ACT_Template_CycleTime(S)"(w91) -> ()
    n196 = Bundle By Name(cluster=w89, "Update Display"=FALSE) -> (w92:T39)
  }
  n197 = flat-sequence {
    frame #0 {
      (unwired) ENUM_ACT_State."Startup" ("State")
      (unwired) ENUM_ACT_Action."No Action" ("Action")
      # "State LIST"
      # "Action LIST"
    }
  }
  n198 = Unbundle By Name(w28) -> ("Steer Refs"=w25:T32[], "Drive Refs"=w13:T32[])
  n199 = for {
    tunnel: w25 -> [w495] mode=indexing
    tunnel: w13 -> [w494] mode=indexing
    n200 = call <vilib>:"WPI_MotorControlDisable.vi"("MotorControlDevRef"=w494) -> ()  [unwired: 9 in, 2 out]
    n201 = call <vilib>:"WPI_MotorControlDisable.vi"("MotorControlDevRef"=w495) -> ()  [unwired: 9 in, 2 out]
  }
